vi "Main.vi"() -> ()   [LabVIEW 2013]
uses:
  ViewCtl.ctl
  GlobalV.vi
panel:
  in  "退出":bool
  in  "ViewCtl":T1
  in  "选项":enum32{"自产包装", "外购机BSJ包装", "出货", "大箱条码打印"}(tab)
  in  "料号":string
  in  "Adress":string caption="发货地址"
  in  "产品型号":u16(ring) items=["9068", "8068", "TRG80-68", "TRG80-68AW", "TRG90-68", "TRG90-68C", "TRG90-68G", "TRG90-68W", "TRG90-68CG", "TRG90-68CW", "TRG90-68GW", "TRG90-68S", "TRG80-89", "TRG90-88", "TRG90-88B", "TRG90-88C", "TRG90-88D", "TRG90-88W", "TRG90-88BW", "TRG90-88CW", "TRG90-88DW", "TRG90-03", "TRG90-03B", "TRG90-03C", "TRG90-03D", "TRG90-03E", "TRG90-03F", "TRG80-03", "TRG80-03B", "TRG80-03D"]
  out "整箱数量":string
  in  "允许未满封箱？":bool=TRUE
  in  "产品条码":string
  in  "手动装箱":bool
  in  "删除单个条码":bool
  in  "包装箱内数据":i32(listbox)
  in  "产品类别":u16(ring) items=["带卡产品", "非带卡产品"]
  in  "扫描方式":u16(ring) caption="扫描入库方式" items=["单个产品码扫描", "整箱产品码扫描"]
  out "记录导入结果":string
  in  "客户地址":string caption="发货地址"
  in  "能未满封箱？":bool=TRUE caption="允许未满封箱？"
  in  "SN码":string caption="产品条码"
  in  "人工封箱":bool
  in  "删除单个数据":bool
  in  "数据导入":bool
  in  "BSJ型号":u16(ring) caption="产品型号" items=["90-18", "90-68"]
  out "一箱数量":string
  in  "BSJ产品记录":i32(listbox)
  in  "地址":string
  in  "导出":bool
  in  "型号":u16(ring) caption="产品型号" items=["90-18", "9068"]
  in  "出货地址":string
  in  "手动出货":bool
  in  "包装箱条码":string
  in  "设定出货数量":string
  in  "出货方式":bool=TRUE
  in  "箱内产品信息":i32(listbox)
  in  "结束时间":timestamp=timestamp(3579818400.015625 s since 1904-01-01) format="%<%H:%M:%S\n%Y/%m/%d>T"
  in  "开始时间":timestamp=timestamp(3579213600.234375 s since 1904-01-01) format="%<%H:%M:%S\n%Y/%m/%d>T"
  in  "导出方式":u16(ring)=1 items=["发货地址", "包装时间", "地址和包装时间"]
  in  "产品种类":u16(ring) items=["外购带卡", "外购不带卡", "自产"]
  in  "类别":u16(ring) caption="产品种类" items=["外购", "自产"]
  in  "PModel":u16(ring) caption="产品型号" items=["9068", "8068", "TRG80-68", "TRG80-68AW", "TRG90-68", "TRG90-68C", "TRG90-68G", "TRG90-68W", "TRG90-68CG", "TRG90-68CW", "TRG90-68GW", "TRG90-68S", "TRG80-89", "TRG90-88", "TRG90-88B", "TRG90-88C", "TRG90-88D", "TRG90-88W", "TRG90-88BW", "TRG90-88CW", "TRG90-88DW", "TRG90-03", "TRG90-03B", "TRG90-03C", "TRG90-03D", "TRG90-03E", "TRG90-03F", "TRG80-03", "TRG80-03B", "TRG80-03D"]
  out "当前大箱内数量":u32
  in  "清空":bool
  in  "条码":string caption="中箱条码"
  out "大箱内产品":string
  in  "设定大箱总数":i32 step=1
  in  "手动计数打印？":bool=TRUE
  in  "手动打印":bool
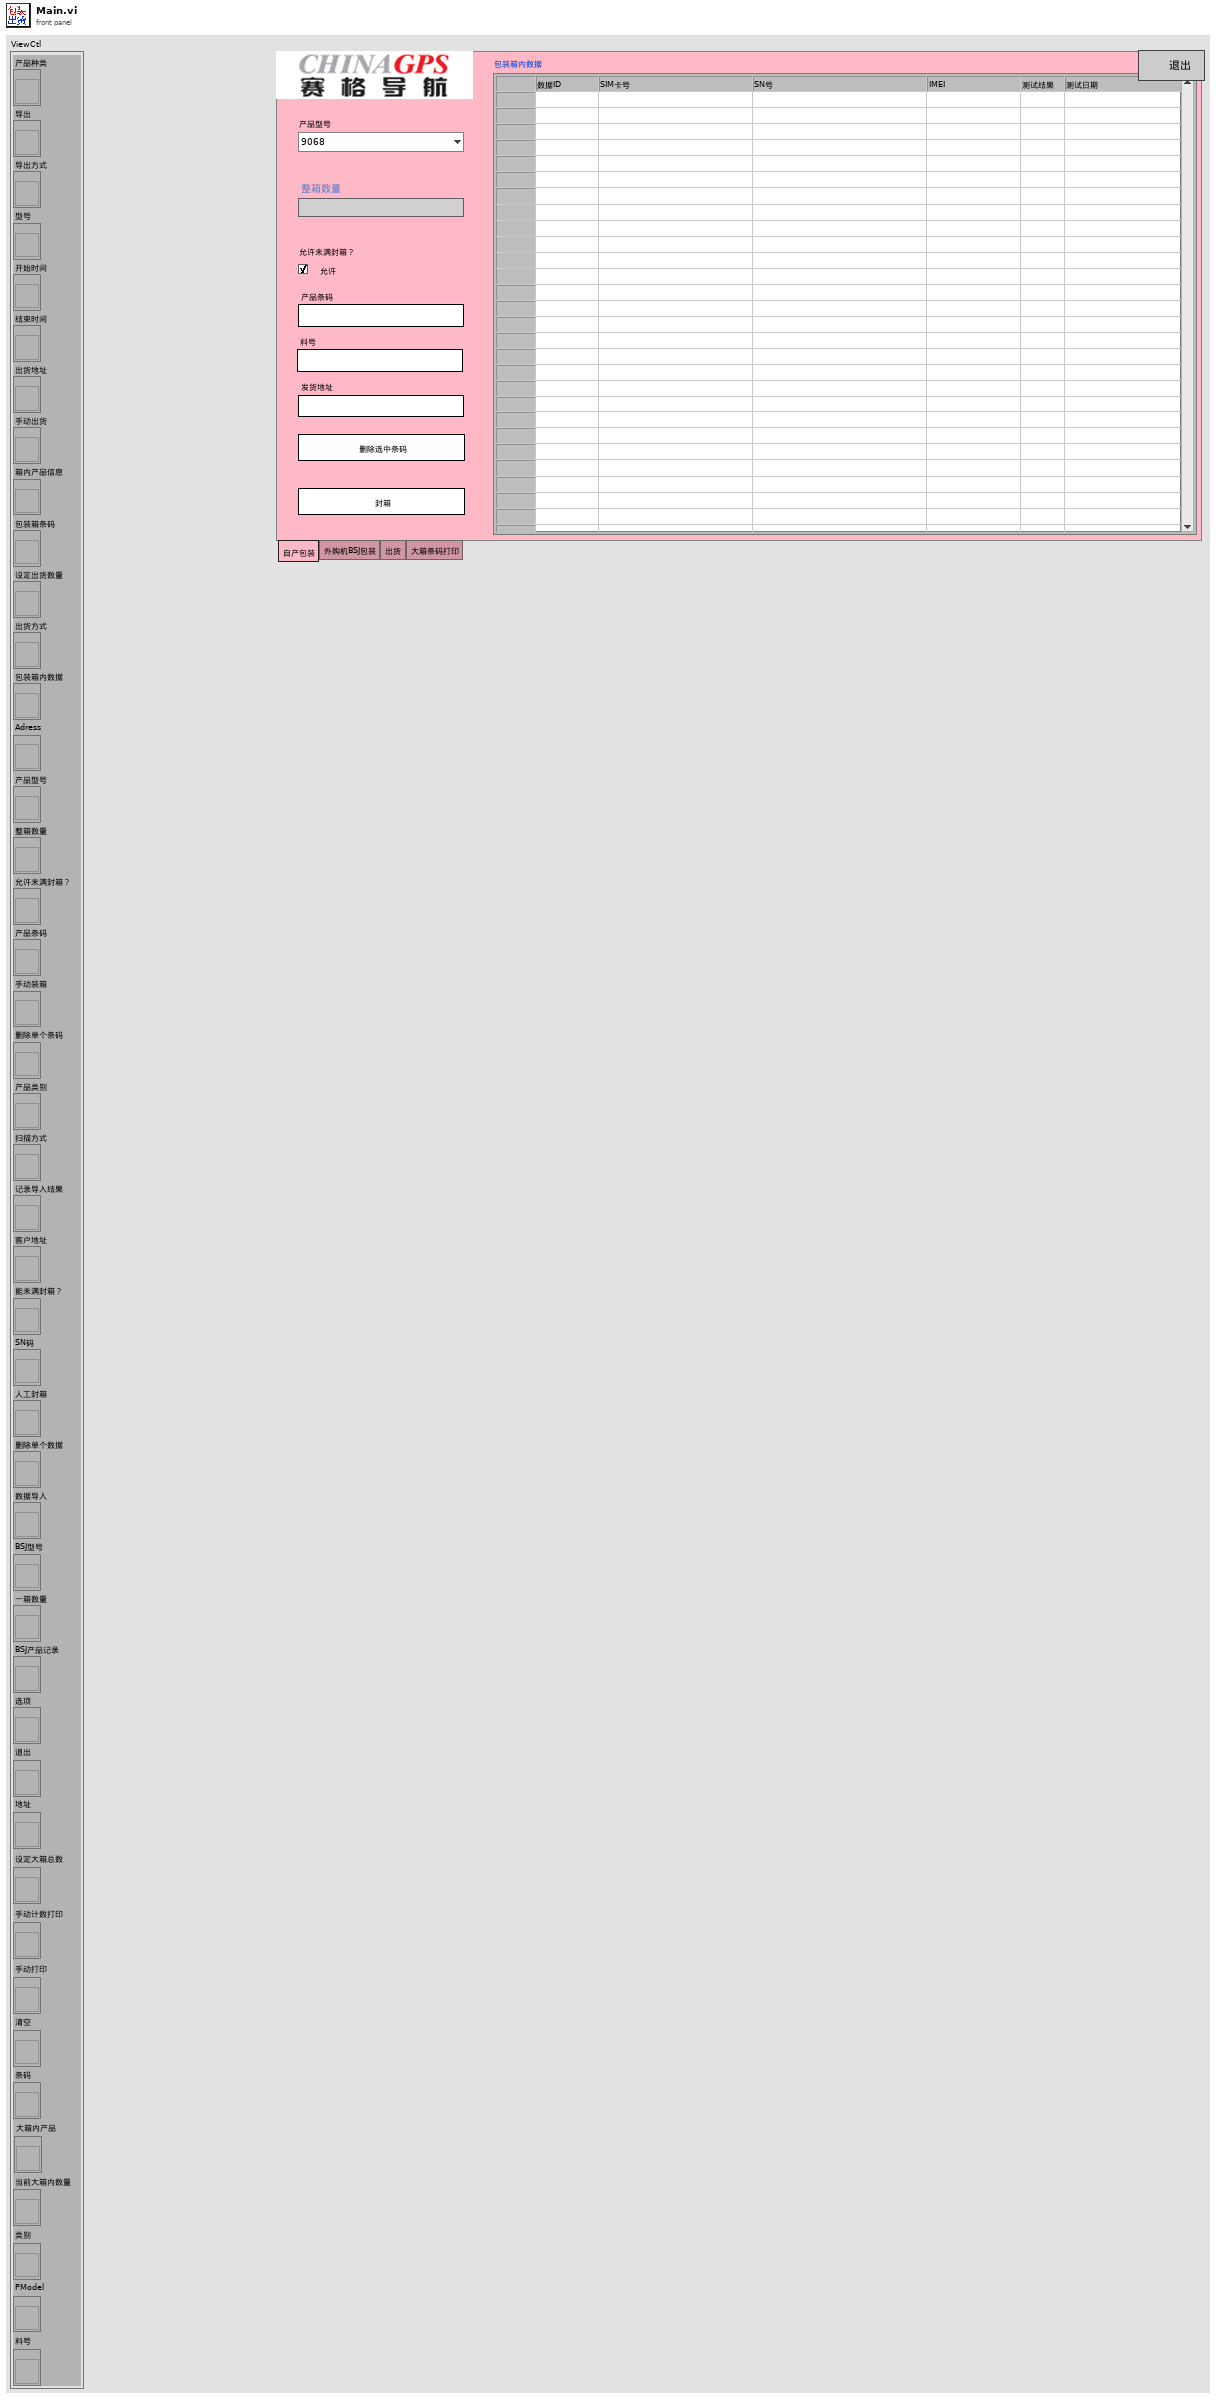
[diagram p1: front panel]
types:
  T1 = typedef "ViewCtl.ctl" = cluster{"产品种类":refnum<vi>, "导出":refnum<vi>, "导出方式":refnum<vi>, "型号":refnum<vi>, "开始时间":refnum<vi>, "结束时间":refnum<vi>, "出货地址":refnum<vi>, "手动出货":refnum<vi>, "箱内产品信息":refnum<vi>, "包装箱条码":refnum<vi>, "设定出货数量":refnum<vi>, "出货方式":refnum<vi>, "包装箱内数据":refnum<vi>, "Adress":refnum<vi>, "产品型号":refnum<vi>, "整箱数量":refnum<vi>, "允许未满封箱？":refnum<vi>, "产品条码":refnum<vi>, "手动装箱":refnum<vi>, "删除单个条码":refnum<vi>, "产品类别":refnum<vi>, "扫描方式":refnum<vi>, "记录导入结果":refnum<vi>, "客户地址":refnum<vi>, "能未满封箱？":refnum<vi>, "SN码":refnum<vi>, "人工封箱":refnum<vi>, "删除单个数据":refnum<vi>, "数据导入":refnum<vi>, "BSJ型号":refnum<vi>, "一箱数量":refnum<vi>, "BSJ产品记录":refnum<vi>, "选项":refnum<vi>, "退出":refnum<vi>, "地址":refnum<vi>, "设定大箱总数":refnum<vi>, "手动计数打印":refnum<vi>, "手动打印":refnum<vi>, "清空":refnum<vi>, "条码":refnum<vi>, "大箱内产品":refnum<vi>, "当前大箱内数量":refnum<vi>, "类别":refnum<vi>, "PModel":refnum<vi>, "料号":refnum<vi>}
  T2 = cluster{"事件注册引用句柄":refnum<event-registration>, "事件注册引用句柄":refnum<event-registration>}
  T3 = enum8{"Enabled", "Disabled", "Disabled and Grayed Out"}
  T4 = typedef "LVRowAndColumnUnsignedTypeDef.ctl" = cluster{"Row":u32, "Column":u32}
  T5 = enum32{"invalid app kind", "Development System", "Run Time System", "Student Edition", "Embedded LabVIEW", "Evaluation", "Custom"}
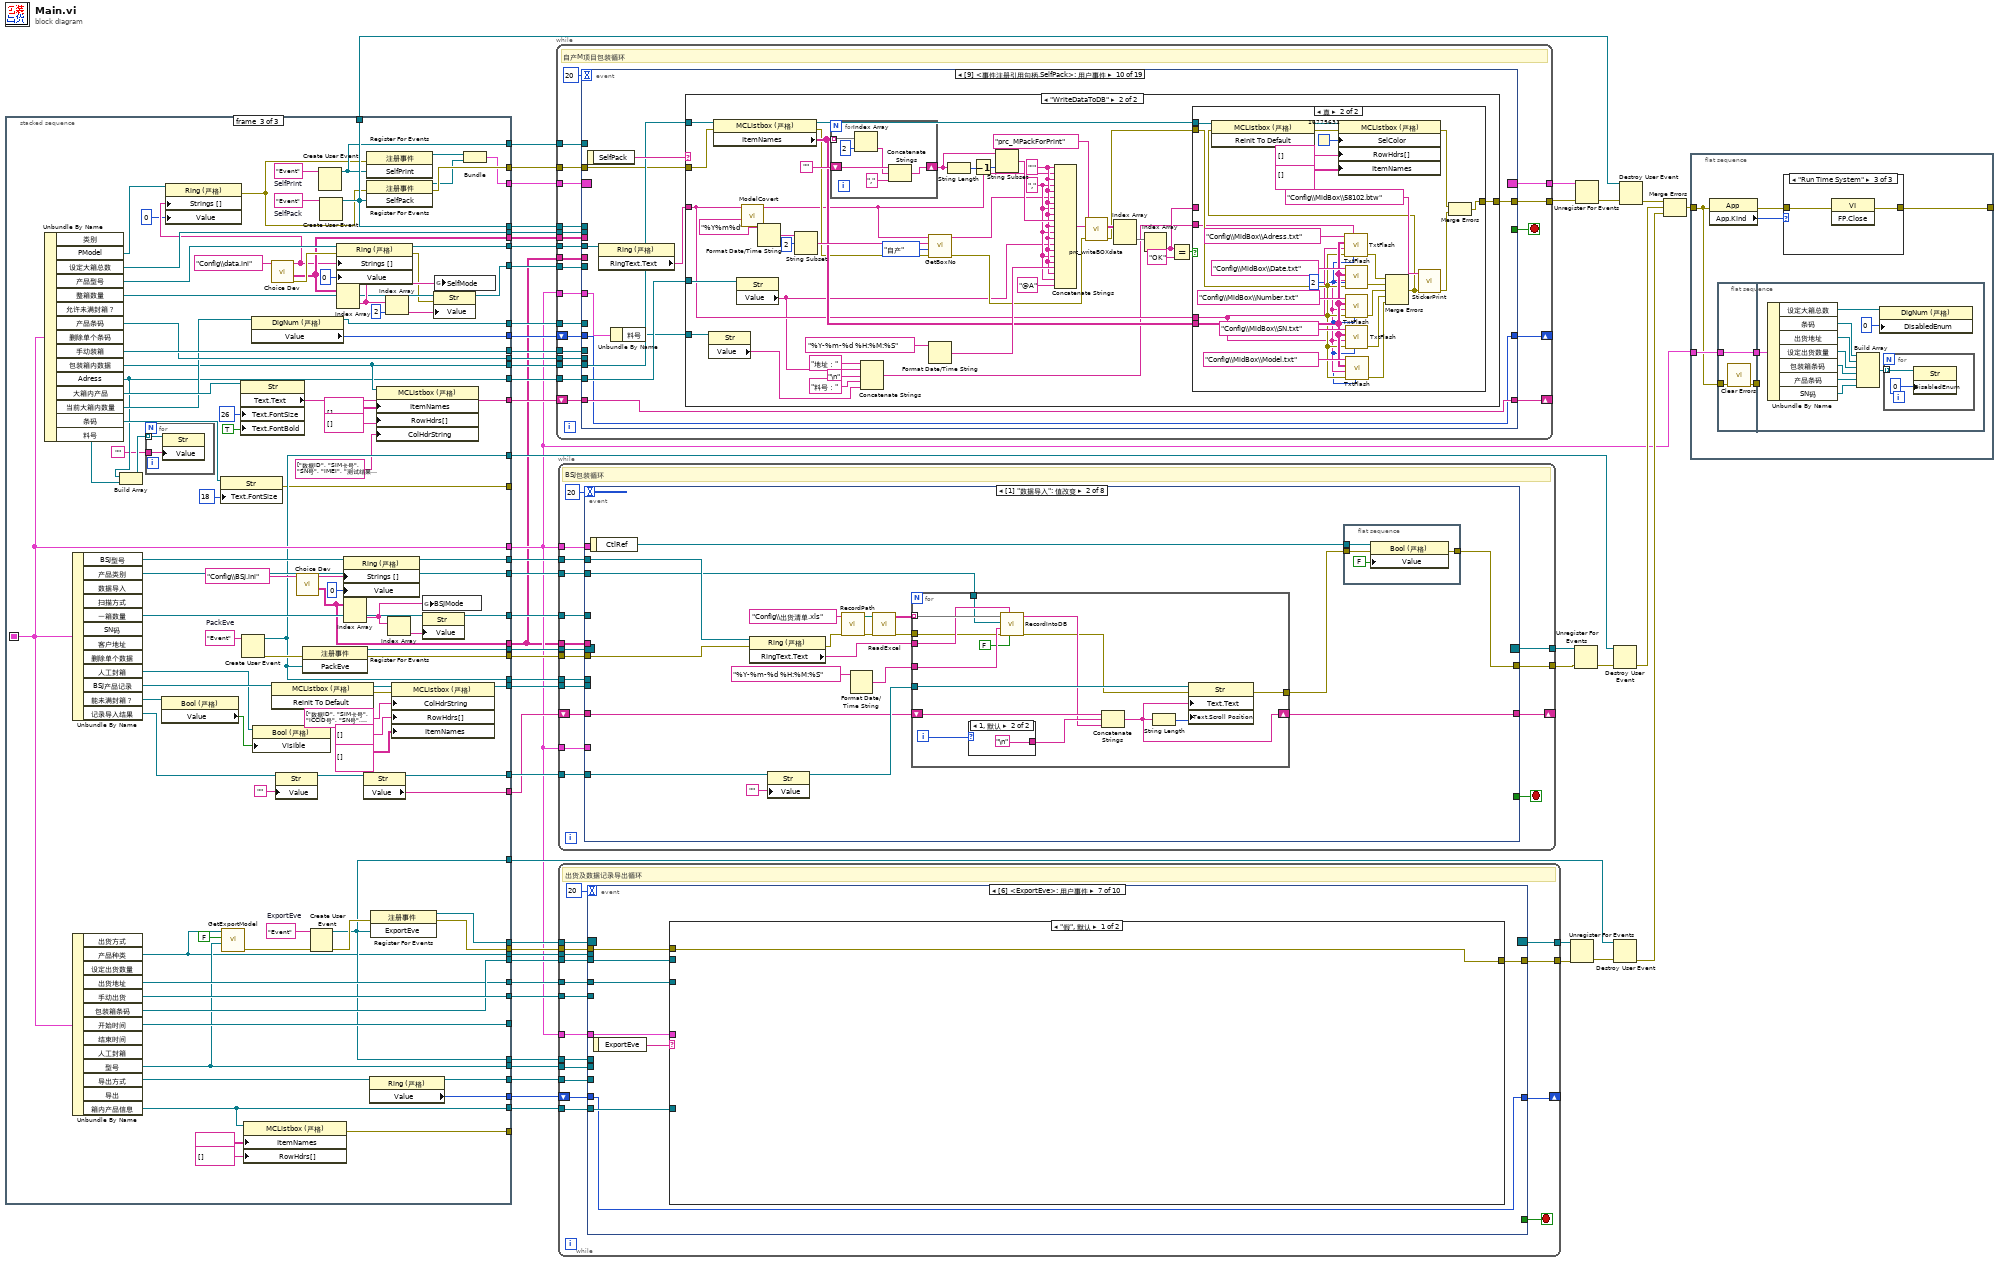
[diagram p0: block diagram]
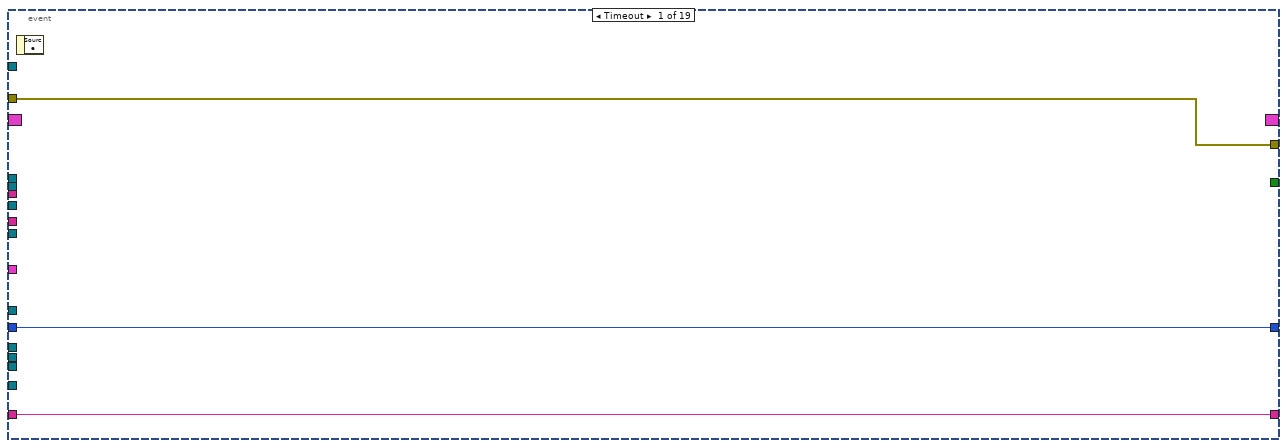
[diagram p4: hidden frame]
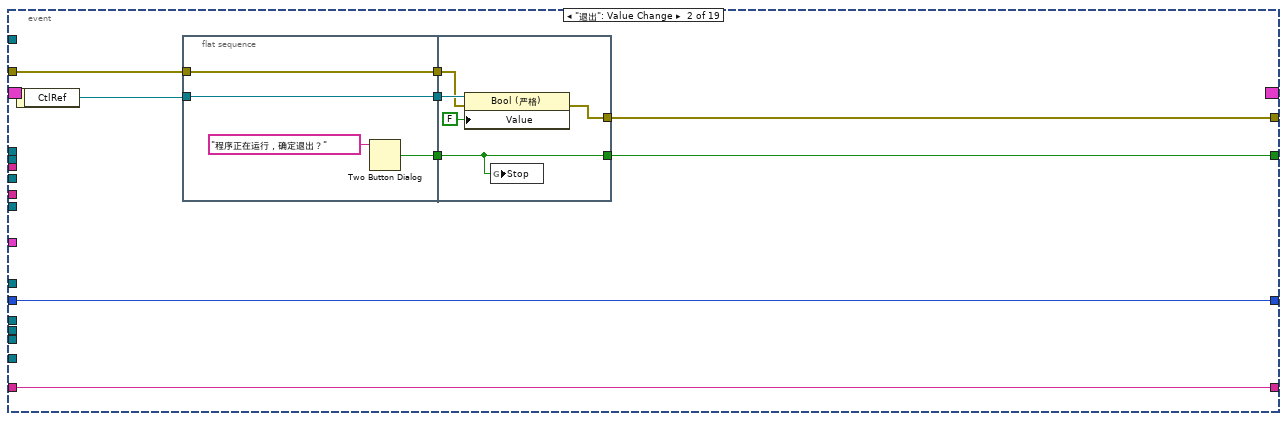
[diagram p5: hidden frame]
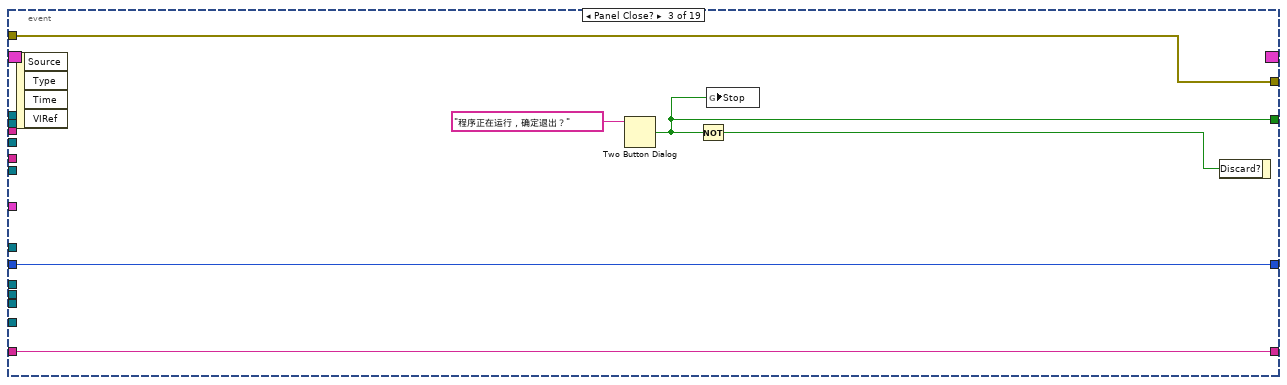
[diagram p6: hidden frame]
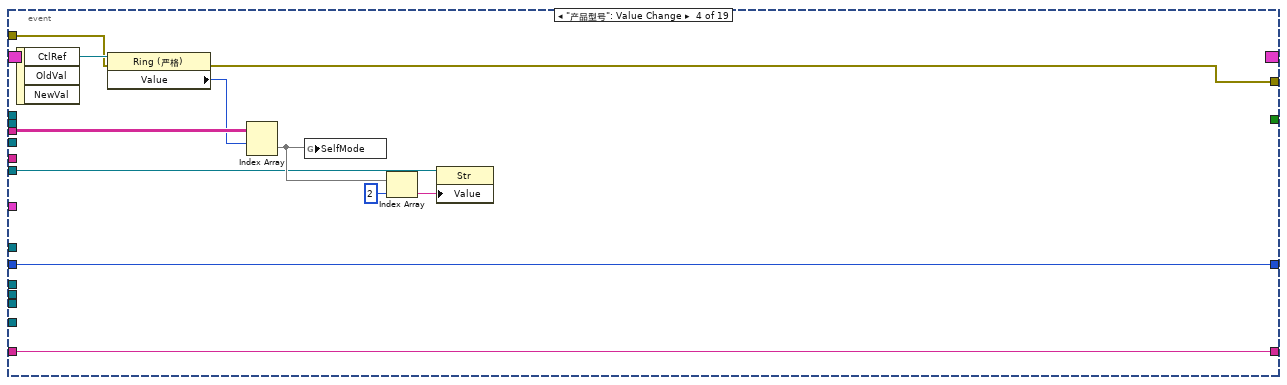
[diagram p7: hidden frame]
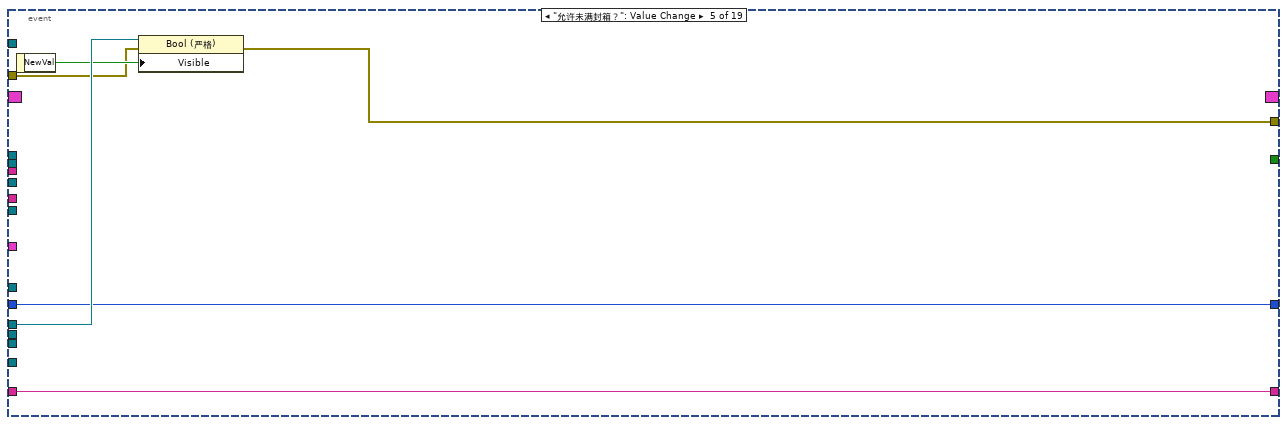
[diagram p8: hidden frame]
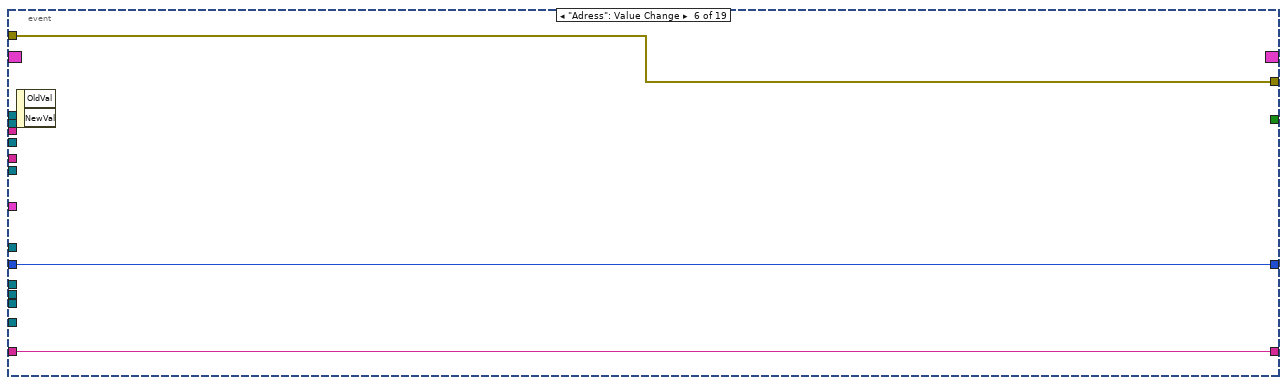
[diagram p9: hidden frame]
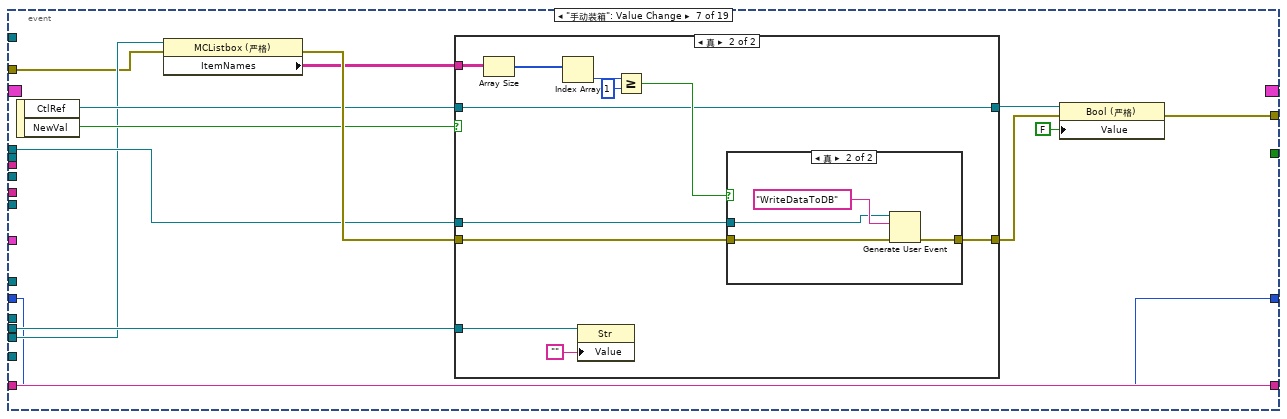
[diagram p10: hidden frame]
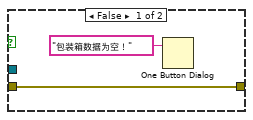
[diagram p12: hidden frame]
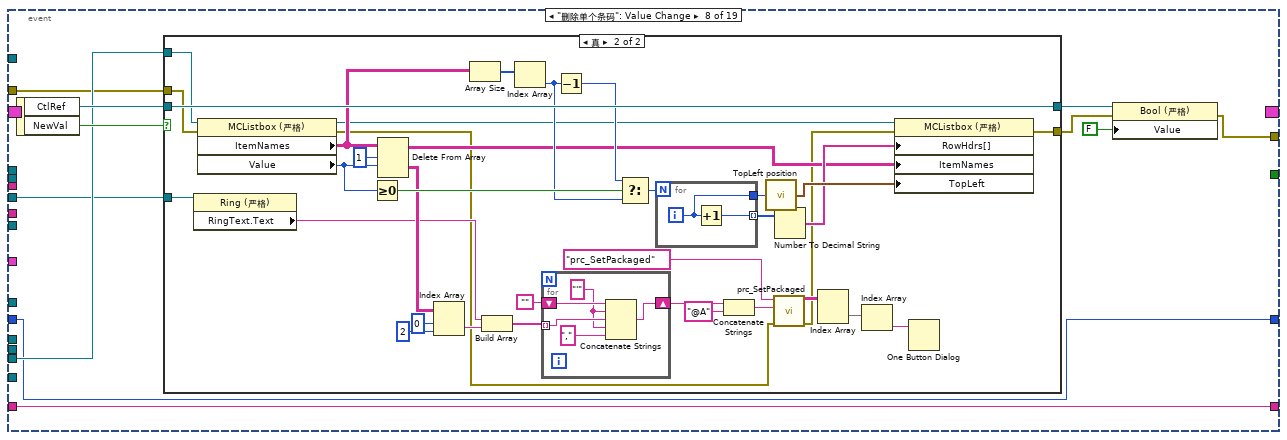
[diagram p13: hidden frame]
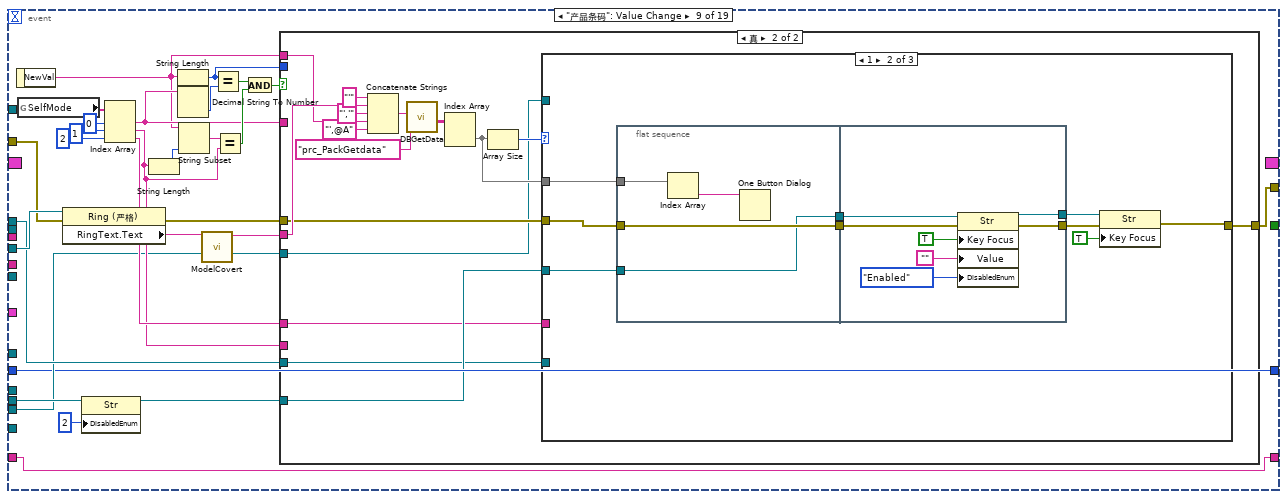
[diagram p15: hidden frame]
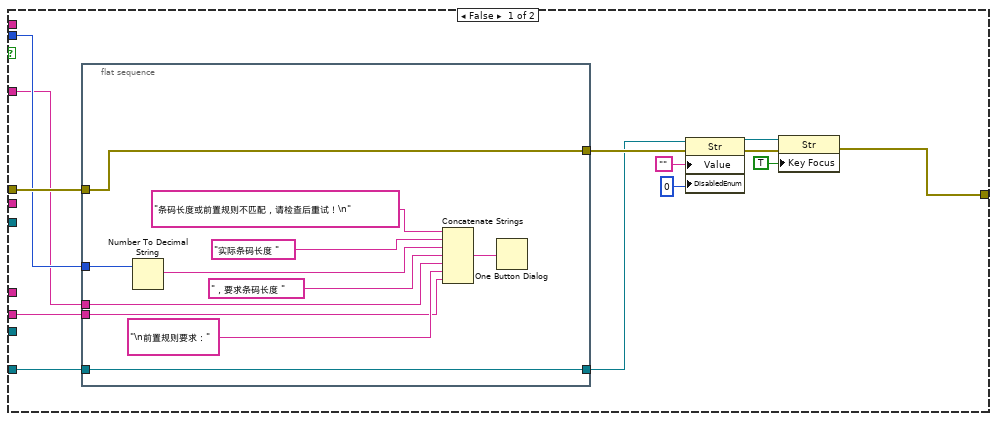
[diagram p16: hidden frame]
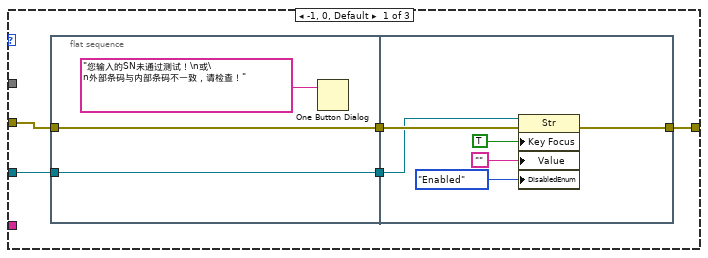
[diagram p17: hidden frame]
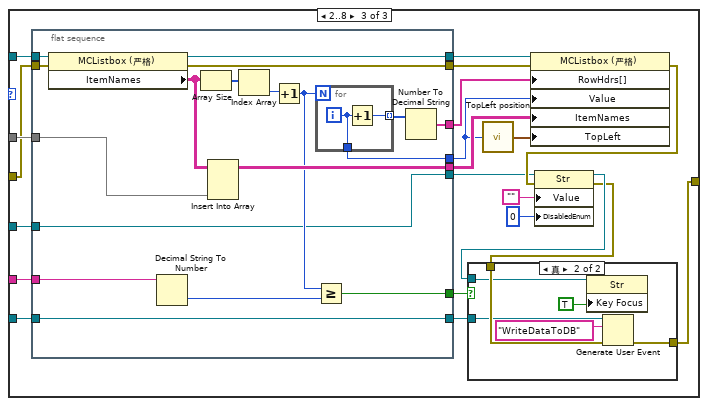
[diagram p18: hidden frame]
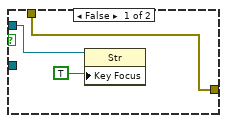
[diagram p19: hidden frame]
diagram:
  n1 = stacked-sequence {
    seq-local: [_ w57 _] -> [_ _ w175]
    tunnel: [_ _ w188] -> w45
    tunnel: [_ _ w185] -> w53
    tunnel: [_ _ w181] -> w52
    tunnel: [_ _ w180] -> w51
    tunnel: [_ _ w179] -> w50
    tunnel: [_ _ w178] -> w1
    tunnel: [_ _ w177] -> w49
    tunnel: [_ _ w176] -> w48
    tunnel: [_ _ w175] -> w3
    tunnel: [_ _ w174] -> w47
    tunnel: [_ _ w146] -> w46
    tunnel: [_ _ w173] -> w44
    tunnel: [_ _ w118] -> w43
    tunnel: [_ _ w171] -> w42
    tunnel: [_ _ w169] -> w41
    tunnel: [_ _ w117] -> w40
    tunnel: [_ _ w168] -> w39
    tunnel: [_ _ w145] -> w38
    tunnel: [_ _ w127] -> w37
    tunnel: [_ _ w167] -> w36
    tunnel: [_ _ w165] -> w35
    tunnel: [_ _ w164] -> w34
    tunnel: [_ _ w163] -> _
    tunnel: [_ _ w153] -> w33
    tunnel: [_ _ w152] -> w32
    tunnel: [_ _ w134] -> w31
    tunnel: [_ _ w147] -> w30
    tunnel: [_ _ w150] -> w29
    tunnel: [_ _ w125] -> w28
    tunnel: [_ _ w149] -> w27
    tunnel: [_ _ w111] -> w26
    tunnel: [_ _ w148] -> w22
    tunnel: [_ _ w147] -> w17
    tunnel: [_ _ w146] -> w15
    tunnel: [_ _ w145] -> w13
    tunnel: [_ _ w143] -> w8
    tunnel: [_ _ w141] -> w7
    tunnel: [_ _ w138] -> w6
    tunnel: [_ _ w133] -> w5
    tunnel: [_ _ w132] -> w4
    tunnel: [_ _ w129] -> _
    tunnel: [_ _ w128] -> w2
    tunnel: [_ _ w120] -> _
    frame #0 {
      n2 = global write "GlobalV.vi" "Stop"(FALSE ("Stop")) -> ()
    }
    frame #1 {
      n3 = invoke class="VI" method="Default Vals.Reinit All"() -> (error out=w58:errorcluster)  [unwired: 3 in, 2 out]
      n4 = flat-sequence {
        tunnel: w58 -> [_]
        tunnel: [w73] -> w57
        frame #0 {
          n5 = control-ref of="箱内产品信息"() -> (w98:refnum<vi>)
          n6 = control-ref of="包装箱内数据"() -> (w94:refnum<vi>)
          n7 = control-ref of="BSJ产品记录"() -> (w75:refnum<vi>)
          n8 = control-ref of="选项"() -> (w74:refnum<vi>)
          n9 = control-ref of="产品种类"() -> (w106:refnum<vi>)
          n10 = control-ref of="导出方式"() -> (w104:refnum<vi>)
          n11 = control-ref of="型号"() -> (w103:refnum<vi>)
          n12 = control-ref of="开始时间"() -> (w102:refnum<vi>)
          n13 = control-ref of="结束时间"() -> (w101:refnum<vi>)
          n14 = control-ref of="产品型号"() -> (w92:refnum<vi>)
          n15 = control-ref of="产品类别"() -> (w86:refnum<vi>)
          n16 = control-ref of="扫描方式"() -> (w85:refnum<vi>)
          n17 = control-ref of="BSJ型号"() -> (w77:refnum<vi>)
          n18 = control-ref of="类别"() -> (w63:refnum<vi>)
          n19 = control-ref of="PModel"() -> (w62:refnum<vi>)
          n20 = control-ref of="出货地址"() -> (w100:refnum<vi>)
          n21 = control-ref of="包装箱条码"() -> (w97:refnum<vi>)
          n22 = control-ref of="设定出货数量"() -> (w96:refnum<vi>)
          n23 = control-ref of="Adress"() -> (w93:refnum<vi>)
          n24 = control-ref of="整箱数量"() -> (w91:refnum<vi>)
          n25 = control-ref of="产品条码"() -> (w89:refnum<vi>)
          n26 = control-ref of="记录导入结果"() -> (w84:refnum<vi>)
          n27 = control-ref of="客户地址"() -> (w83:refnum<vi>)
          n28 = control-ref of="SN码"() -> (w81:refnum<vi>)
          n29 = control-ref of="一箱数量"() -> (w76:refnum<vi>)
          n30 = control-ref of="地址"() -> (w71:refnum<vi>)
          n31 = control-ref of="条码"() -> (w66:refnum<vi>)
          n32 = control-ref of="大箱内产品"() -> (w65:refnum<vi>)
          n33 = control-ref of="料号"() -> (w61:refnum<vi>)
          n34 = control-ref of="导出"() -> (w105:refnum<vi>)
          n35 = control-ref of="手动出货"() -> (w99:refnum<vi>)
          n36 = control-ref of="出货方式"() -> (w95:refnum<vi>)
          n37 = control-ref of="允许未满封箱？"() -> (w90:refnum<vi>)
          n38 = control-ref of="手动装箱"() -> (w88:refnum<vi>)
          n39 = control-ref of="删除单个条码"() -> (w87:refnum<vi>)
          n40 = control-ref of="能未满封箱？"() -> (w82:refnum<vi>)
          n41 = control-ref of="人工封箱"() -> (w80:refnum<vi>)
          n42 = control-ref of="删除单个数据"() -> (w79:refnum<vi>)
          n43 = control-ref of="数据导入"() -> (w78:refnum<vi>)
          n44 = control-ref of="退出"() -> (w72:refnum<vi>)
          n45 = control-ref of="设定大箱总数"() -> (w70:refnum<vi>)
          n46 = control-ref of="手动计数打印？"() -> (w69:refnum<vi>)
          n47 = control-ref of="手动打印"() -> (w68:refnum<vi>)
          n48 = control-ref of="清空"() -> (w67:refnum<vi>)
          n49 = control-ref of="当前大箱内数量"() -> (w64:refnum<vi>)
          n50 = Bundle By Name(cluster="ViewCtl", "产品种类"=w106, "导出"=w105, "导出方式"=w104, "型号"=w103, "开始时间"=w102, "结束时间"=w101, "出货地址"=w100, "手动出货"=w99, "箱内产品信息"=w98, "包装箱条码"=w97, "设定出货数量"=w96, "出货方式"=w95, "包装箱内数据"=w94, "Adress"=w93, "产品型号"=w92, "整箱数量"=w91, "允许未满封箱？"=w90, "产品条码"=w89, "手动装箱"=w88, "删除单个条码"=w87, "产品类别"=w86, "扫描方式"=w85, "记录导入结果"=w84, "客户地址"=w83, "能未满封箱？"=w82, "SN码"=w81, "人工封箱"=w80, "删除单个数据"=w79, "数据导入"=w78, "BSJ型号"=w77, "一箱数量"=w76, "BSJ产品记录"=w75, "选项"=w74, "退出"=w72, "地址"=w71, "设定大箱总数"=w70, "手动计数打印"=w69, "手动打印"=w68, "清空"=w67, "条码"=w66, "大箱内产品"=w65, "当前大箱内数量"=w64, "类别"=w63, "PModel"=w62, "料号"=w61) -> (w73:T1)
        }
      }
      n51 = Unbundle By Name(w57) -> ("选项"=w56:refnum<vi>)
      n52 = property class="TabCtl (严格)"(reference=w56) -> ("Pages"=w55:refnum<vi>[])  [unwired: 1 in, 2 out]
      n53 = for {
        tunnel: w55 -> [w60] mode=indexing
        n54 = property class="Page"(reference=w60, "PageEnb"=2) -> ()  [unwired: 1 in, 2 out]
      }
    }
    frame #2 {
      w137 = "Event"  # SelfPrint
      w151 = "Event"  # SelfPack
      w172 = "Event"  # ExportEve
      w187 = "Event"  # PackEve
      n55 = Unbundle By Name(w175) -> ("PModel"=w115:refnum<vi>, "设定大箱总数"=w138:refnum<vi>, "产品型号"=w161:refnum<vi>, "整箱数量"=w158:refnum<vi>, "产品条码"=w150:refnum<vi>, "手动装箱"=w152:refnum<vi>, "包装箱内数据"=w125:refnum<vi>, "Adress"=w111:refnum<vi>, "大箱内产品"=w144:refnum<vi>, "当前大箱内数量"=w142:refnum<vi>, "条码"=w131:refnum<vi>, "料号"=w110:refnum<vi>)  [unwired: 3 out]
      n56 = Unbundle By Name(w175) -> ("BSJ型号"=w203:refnum<vi>, "产品类别"=w174:refnum<vi>, "一箱数量"=w192:refnum<vi>, "人工封箱"=w190:refnum<vi>, "BSJ产品记录"=w200:refnum<vi>, "能未满封箱？"=w191:refnum<vi>, "记录导入结果"=w183:refnum<vi>)  [unwired: 5 out]
      n57 = Unbundle By Name(w175) -> ("产品种类"=w117:refnum<vi>, "出货地址"=w167:refnum<vi>, "手动出货"=w173:refnum<vi>, "包装箱条码"=w168:refnum<vi>, "开始时间"=w163:refnum<vi>, "型号"=w118:refnum<vi>, "导出方式"=w166:refnum<vi>, "箱内产品信息"=w127:refnum<vi>)  [unwired: 5 out]
      n58 = Build Array(w111, w110) -> (w109:refnum<vi>[])
      n59 = for {
        tunnel: w109 -> [w206] mode=indexing
        tunnel: "" -> [w205]
        n60 = property class="Str"(reference=w206, "Value"=w205) -> ()  [unwired: 1 in, 2 out]
      }
      n61 = property class="Bool (严格)"(reference=w191) -> ("Value"=w189:bool)  [unwired: 1 in, 2 out]
      n62 = property class="Str"(reference=w131, "Text.FontSize"=u32 18 ("文本.字体:字号")) -> (error out=w129:errorcluster)  [unwired: 1 in, 1 out]
      n63 = call "GetExportModel.vi"("型号"=w118, "Debug"=FALSE, "产品类型"=w117) -> ("error out"=w116:errorcluster)  [unwired: 8 in]
      n64 = property class="Str"(reference=w144, "Text.FontSize"=u32 26 ("文本.字体:字号"), "Text.FontBold"=TRUE) -> ("Text.Text"=w143:string)  [unwired: 1 in, 2 out]
      n65 = Create User Event(user event datatype=w187) -> (user event=w146:refnum<user-event>, error out=w186:errorcluster)  [unwired: 1 in]
      n66 = property class="MCListbox (严格)"(reference=w127, "ItemNames"=string[][] [] ("项名"), "RowHdrs[]"=string[] [] ("行首字符串[]")) -> (error out=w120:errorcluster)  [unwired: 1 in, 1 out]
      n67 = property class="DigNum (严格)"(reference=w142) -> (reference out=w132:refnum<vi>, "Value"=w141:u32)  [unwired: 1 in, 1 out]
      n68 = property class="Bool (严格)"(reference=w190, "Visible"=w189) -> ()  [unwired: 1 in, 2 out]
      n69 = call "Choice Dev.vi"("Path"="Config\\data.ini") -> ("error out"=w155:errorcluster, "data"=w153:string[][], "model"=w114:string[])  [unwired: 7 in]
      n70 = property class="Ring (严格)"(reference=w115, "Strings []"=w114, "Value"=u16 0 ("值")) -> (error out=w112:errorcluster)  [unwired: 1 in, 1 out]
      n71 = invoke class="MCListbox (严格)" method="Reinit To Default"(reference=w200) -> (reference out=w199:refnum<vi>, error out=w195:errorcluster)  [unwired: 2 in, 1 out]
      n72 = property class="Str"(reference=w183, "Value"="") -> (reference out=w182:refnum<vi>)  [unwired: 1 in, 1 out]
      n73 = call "Choice Dev.vi"("Path"="Config\\BSJ.ini") -> ("data"=w178:string[][], "model"=w202:string[])  [unwired: 7 in, 1 out]
      n74 = register-events(error in=w186, w146) -> (reference out=w185:refnum<event-registration>, error out=w176:errorcluster)  [unwired: 1 in]
      n75 = Create User Event(user event datatype=w172, error in=w116) -> (user event=w145:refnum<user-event>, error out=w170:errorcluster)
      n76 = Create User Event(user event datatype=w137) -> (user event=w133:refnum<user-event>)  [unwired: 1 in, 1 out]
      n77 = Create User Event(user event datatype=w151) -> (user event=w147:refnum<user-event>)  [unwired: 1 in, 1 out]
      n78 = property class="Ring (严格)"(reference=w161, error in=w155, "Strings []"=w114, "Value"=u16 0 ("值")) -> (reference out=w149:refnum<vi>, error out=w154:errorcluster)
      n79 = Index Array(array=w153) -> (element=w159:string[])  [unwired: 2 in]
      n80 = property class="Ring (严格)"(reference=w203, "Strings []"=w202, "Value"=u16 0 ("值")) -> (reference out=w179:refnum<vi>)  [unwired: 1 in, 1 out]
      n81 = Index Array(array=w178) -> (element=w194:string[])  [unwired: 2 in]
      n82 = property class="Str"(reference=w182) -> (reference out=w181:refnum<vi>, "Value"=w180:string)  [unwired: 1 in, 1 out]
      n83 = register-events(error in=w112, w133) -> (reference out=w136:refnum<event-registration>)  [unwired: 1 in, 1 out]
      n84 = register-events(error in=w112, w147) -> (reference out=w135:refnum<event-registration>, error out=w148:errorcluster)  [unwired: 1 in]
      n85 = property class="Ring (严格)"(reference=w166) -> (reference out=w164:refnum<vi>, "Value"=w165:u16)  [unwired: 1 in, 1 out]
      n86 = register-events(error in=w170, w145) -> (reference out=w171:refnum<event-registration>, error out=w169:errorcluster)  [unwired: 1 in]
      n87 = property class="MCListbox (严格)"(reference=w125, "ItemNames"=string[][] [] ("项名"), "RowHdrs[]"=string[] [] ("行首字符串[]"), "ColHdrString"=string[] ["数据ID", "SIM卡号", "SN号", "IMEI", "测试结果", "测试日期"]) -> ()  [unwired: 1 in, 2 out]
      n88 = Index Array(array=w159, index=2 ("索引")) -> (element=w157:string)
      n89 = Index Array(array=w194) -> (element=w193:string)  [unwired: 1 in]
      n90 = property class="MCListbox (严格)"(reference=w199, error in=w195, "ColHdrString"=string[] ["数据ID", "SIM卡号", "ICCID号", "SN号", "导入日期"], "RowHdrs[]"=string[] [] ("行首字符串[]"), "ItemNames"=string[][] [] ("项名")) -> (reference out=w188:refnum<vi>)  [unwired: 1 out]
      n91 = global write "GlobalV.vi" "BSJMode"(w194) -> ()
      n92 = property class="Str"(reference=w192, "Value"=w193) -> (reference out=w177:refnum<vi>)  [unwired: 1 in, 1 out]
      n93 = property class="Str"(reference=w158, error in=w154, "Value"=w157) -> (reference out=w128:refnum<vi>)  [unwired: 1 out]
      n94 = global write "GlobalV.vi" "SelfMode"(w159) -> ()
      n95 = Bundle("事件注册引用句柄"=w136, "事件注册引用句柄"=w135) -> (w134:T2)  [unwired: 1 in]
    }
  }
  n96 = while {
    tunnel: w33 -> [w227]
    tunnel: w32 -> [w226]
    tunnel: w31 -> [w225]
    tunnel: w30 -> [w224]
    tunnel: w29 -> [w223]
    tunnel: w28 -> [w222]
    tunnel: w27 -> [w221]
    tunnel: w26 -> [w220]
    tunnel: [w219] -> w25
    tunnel: w22 -> [w218]
    tunnel: [w217] -> w21
    tunnel: w3 -> [w216]
    shift-right: [w214] -> _
    shift-left: w8 -> [w215]
    shift-right: [w212] -> _
    shift-left: w7 -> [w213]
    tunnel: w6 -> [w211]
    tunnel: w5 -> [w210]
    tunnel: w4 -> [w209]
    tunnel: w2 -> [w208]
    tunnel: w1 -> [w207]
    stop <- w228 stop-if-true
    # "自产M项目包装循环"
    n97 = event shown="[9] <事件注册引用句柄.SelfPack>: 用户事件" {
      selector: w225 -> [_ _ _ _ _ _ _ _ _ _ _ _ _ _ _ _ _ _ _]
      dyn-events: [_ _ _ _ _ _ _ _ _ _ _ _ _ _ _ _ _ _ _] -> w219
      timeout: 20 -> [_ _ _ _ _ _ _ _ _ _ _ _ _ _ _ _ _ _ _]
      tunnel: [_ w238 w254 _ _ _ _ _ _ _ _ _ _ _ _ _ _ _ _] -> w228
      tunnel: w227 -> [_ _ _ w266 _ _ _ _ _ _ _ _ _ _ _ _ _ w1126 _]
      tunnel: w226 -> [_ _ _ _ w273 _ _ _ _ _ _ _ _ _ _ _ _ _ _]
      tunnel: w224 -> [_ _ _ _ _ _ w283 _ w376 _ _ _ _ _ _ _ _ _ _]
      tunnel: w223 -> [_ _ _ _ _ _ w282 _ w381 _ _ _ _ _ _ _ _ _ _]
      tunnel: w222 -> [_ _ _ _ _ _ w281 w316 w372 w526 _ _ _ _ _ _ _ _ _]
      tunnel: w221 -> [_ _ _ _ _ _ _ w315 w378 w525 _ _ _ _ _ _ _ _ _]
      tunnel: w220 -> [_ _ _ _ _ _ _ _ _ w523 _ _ _ _ _ _ _ _ _]
      tunnel: w218 -> [w232 w236 w253 w264 w271 w276 w280 w313 w371 w522 w608 w752 w796 w805 w1012 w1044 w1098 w1134 w1148]
      tunnel: [w232 w235 w253 w263 w270 w276 w279 w312 w370 w521 w608 w751 w795 w806 w1006 w1043 w1097 w1134 w1148] -> w217
      tunnel: w216 -> [_ _ _ _ _ _ _ _ _ w518 w606 _ w799 w817 _ w1040 w1100 w1131 w1139]
      tunnel: w215 -> [w231 w234 w252 w262 w269 w275 w278 w311 w369 w520 w605 w750 w794 w800 w1011 w1038 w1103 w1133 w1145]
      tunnel: [w231 w234 w252 w262 w269 w275 w278 w311 w369 w520 w605 w750 w794 w807 w1011 w1039 w1103 w1133 w1140] -> w214
      tunnel: w213 -> [w230 w233 w251 w261 w268 w274 w277 w310 w368 w519 w604 w749 w793 w820 w1013 w1037 w1102 w1132 w1144]
      tunnel: [w230 w233 w251 w261 w268 w274 w277 w310 w368 w519 w604 w749 w793 w819 w1013 w1036 w1102 w1132 w1141] -> w212
      tunnel: w211 -> [_ _ _ _ _ _ _ _ _ _ _ _ _ w810 _ _ _ _ _]
      tunnel: w210 -> [_ _ _ _ _ _ _ _ _ _ _ _ _ w811 w1007 _ _ _ _]
      tunnel: w209 -> [_ _ _ _ _ _ _ _ _ _ _ _ _ w808 _ _ _ _ _]
      tunnel: w208 -> [_ _ _ w259 _ _ _ _ _ _ _ _ _ _ _ _ _ _ _]
      tunnel: w207 -> [_ _ _ _ _ _ _ _ _ _ _ _ _ _ _ _ _ w1125 _]
      event Timeout {
        n98 = event-data() -> ()  [unwired: 1 in, 1 out]
      }
      event "退出": Value Change {
        n99 = event-data() -> ("CtlRef"=w239:refnum<vi>)  [unwired: 1 in]
        n100 = flat-sequence {
          tunnel: [w244] -> w241
          tunnel: [w243] -> w240
          tunnel: w239 -> [w243]
          tunnel: [w242] -> w237
          tunnel: w236 -> [w242]
          tunnel: [w248] -> w238
          tunnel: w241 -> [w248]
          tunnel: w240 -> [w250]
          tunnel: w237 -> [w247]
          tunnel: [w246] -> w235
          frame #0 {
            n101 = Two Button Dialog(message="程序正在运行，确定退出？" ("消息")) -> (T button?=w244:bool)  [unwired: 2 in]
          }
          frame #1 {
            n102 = property class="Bool (严格)"(reference=w250, error in=w247, "Value"=FALSE) -> (error out=w246:errorcluster)  [unwired: 1 out]
            n103 = global write "GlobalV.vi" "Stop"(w248) -> ()
          }
        }
      }
      event Panel Close? {
        n104 = event-data() -> ()  [unwired: 1 in, 4 out]
        n105 = Two Button Dialog(message="程序正在运行，确定退出？" ("消息")) -> (T button?=w254:bool)  [unwired: 2 in]
        n106 = Not(x=w254) -> (.not. x?=w255:bool)
        n107 = global write "GlobalV.vi" "Stop"(w254) -> ()
        n108 = event-data("Discard?"=w255) -> ()  [unwired: 1 in, 1 out]
      }
      event "产品型号": Value Change {
        n109 = event-data() -> ("CtlRef"=w267:refnum<vi>)  [unwired: 1 in, 2 out]
        n110 = property class="Ring (严格)"(reference=w267, error in=w264) -> (error out=w263:errorcluster, "Value"=w265:u16)  [unwired: 1 out]
        n111 = Index Array(array=w266, index (row)=w265) -> (element=w260:string[])  [unwired: 1 in]
        n112 = global write "GlobalV.vi" "SelfMode"(w260) -> ()
        n113 = Index Array(array=w260, index=2 ("索引")) -> (element=w258:string)
        n114 = property class="Str"(reference=w259, "Value"=w258) -> ()  [unwired: 1 in, 2 out]
      }
      event "允许未满封箱？": Value Change {
        n115 = event-data() -> ("NewVal"=w272:bool)  [unwired: 1 in]
        n116 = property class="Bool (严格)"(reference=w273, error in=w271, "Visible"=w272) -> (error out=w270:errorcluster)  [unwired: 1 out]
      }
      event "Adress": Value Change {
        n117 = event-data() -> ()  [unwired: 1 in, 2 out]
      }
      event "手动装箱": Value Change {
        n118 = event-data() -> ("CtlRef"=w285:refnum<vi>, "NewVal"=w284:bool)  [unwired: 1 in]
        n119 = property class="MCListbox (严格)"(reference=w281, error in=w280) -> (error out=w289:errorcluster, "ItemNames"=w286:string[][])  [unwired: 1 out]
        n120 = case shown="真" w284 {
          tunnel: w285 -> [w292 w296]
          tunnel: w286 -> [_ w303]
          tunnel: w283 -> [_ w298]
          tunnel: w282 -> [_ w297]
          tunnel: [w292 w296] -> w288
          tunnel: w289 -> [w291 w295]
          tunnel: [w291 w294] -> w290
          frame False {
          }
          frame True {
            n121 = Array Size(array=w303) -> (size(s)=w302:i32[])
            n122 = Index Array(array=w302) -> (element=w301:i32)  [unwired: 1 in]
            n123 = property class="Str"(reference=w297, "Value"="") -> ()  [unwired: 1 in, 2 out]
            n124 = Greater Or Equal?(x=w301, y=1) -> (x >= y?=w299:bool)
            n125 = case shown="真" w299 {
              tunnel: w298 -> [_ w306]
              tunnel: w295 -> [w304 w308]
              tunnel: [w304 w307] -> w294
              frame False {
                n126 = One Button Dialog(message="包装箱数据为空！" ("消息")) -> ()  [unwired: 1 in, 1 out]
              }
              frame True {
                n127 = Generate User Event(user event=w306, event data cluster="WriteDataToDB" ("事件数据"), error in=w308) -> (error out=w307:errorcluster)  [unwired: 1 in, 1 out]
              }
            }
          }
        }
        n128 = property class="Bool (严格)"(reference=w288, error in=w290, "Value"=FALSE ("值")) -> (error out=w279:errorcluster)  [unwired: 1 out]
      }
      event "删除单个条码": Value Change {
        n129 = event-data() -> ("CtlRef"=w318:refnum<vi>, "NewVal"=w317:bool)  [unwired: 1 in]
        n130 = case shown="真" w317 {
          tunnel: w318 -> [w322 w357]
          tunnel: [w322 w357] -> w320
          tunnel: w316 -> [_ w356]
          tunnel: w315 -> [_ w340]
          tunnel: w313 -> [w321 w326]
          tunnel: [w321 w323] -> w314
          frame False {
          }
          frame True {
            n131 = property class="Ring (严格)"(reference=w340) -> ("RingText.Text"=w338:string)  [unwired: 1 in, 2 out]
            n132 = property class="MCListbox (严格)"(reference=w356, error in=w326) -> (reference out=w345:refnum<vi>, error out=w325:errorcluster, "ItemNames"=w354:string[][], "Value"=w352:i32)
            n133 = Greater Or Equal To 0?(x=w352) -> (x >= 0?=w351:bool)
            n134 = Delete From Array(array=w354, length=1 ("长度"), index (row)=w352) -> (deleted portion=w339:string[][], array with subset deleted=w342:string[][])  [unwired: 1 in]
            n135 = Index Array(array=w339, index (row)=0 ("索引 (行)"), index (col)=2 ("禁用的索引 (列)")) -> (element=w337:string)
            n136 = Array Size(array=w354) -> (size(s)=w353:i32[])
            n137 = Build Array(w338, w337) -> (w334:string[])
            n138 = Index Array(array=w353) -> (element=w349:i32)  [unwired: 1 in]
            n139 = for {
              tunnel: w334 -> [w361] mode=indexing
              shift-right: [w358] -> w331
              shift-left: "" -> [w362]
              w360 = "'" ("字符串")
              n140 = Concatenate Strings(w362, w360, w361, w360, "," ("字符串")) -> (w358:string)
            }
            n141 = Decrement(x=w349) -> (x-1=w350:i32)
            n142 = Select(t=w350, s=w351, f=w349) -> (s? t:f=w348:i32)
            n143 = for {
              N: w348 -> [_]
              tunnel: [w364] -> w346 mode=indexing
              tunnel: [w363] -> w347
              i -> [w363]
              n144 = Increment(x=w363) -> (x+1=w364:i32)
            }
            n145 = Concatenate Strings(w331, "@A" ("字符串")) -> (w333:string)
            n146 = call "TopLeft position.vi"("index"=w347) -> ("TopLeft"=w344:T4)
            n147 = call "prc_SetPackaged.vi"("error in"=w325, "string"=w333, "SQL query"="prc_SetPackaged") -> ("error out"=w324:errorcluster, "Array"=w330:string[][])  [unwired: 7 in]
            n148 = Number To Decimal String(number=w346) -> (decimal integer string=w343:string[])  [unwired: 1 in]
            n149 = Index Array(array=w330) -> (element=w329:string[])  [unwired: 2 in]
            n150 = Index Array(array=w329) -> (element=w328:string)  [unwired: 1 in]
            n151 = property class="MCListbox (严格)"(reference=w345, error in=w324, "RowHdrs[]"=w343, "ItemNames"=w342, "TopLeft"=w344) -> (error out=w323:errorcluster)  [unwired: 1 out]
            n152 = One Button Dialog(message=w328) -> ()  [unwired: 1 in, 1 out]
          }
        }
        n153 = property class="Bool (严格)"(reference=w320, error in=w314, "Value"=FALSE ("值")) -> (error out=w312:errorcluster)  [unwired: 1 out]
      }
      event "产品条码": Value Change {
        n154 = event-data() -> ("NewVal"=w367:string)  [unwired: 1 in]
        n155 = global read "GlobalV.vi" "SelfMode"() -> (w391:string[])
        n156 = property class="Ring (严格)"(reference=w378, error in=w371) -> (error out=w392:errorcluster, "RingText.Text"=w366:string)  [unwired: 1 out]
        n157 = property class="Str"(reference=w381, "DisabledEnum"=2) -> (reference out=w379:refnum<vi>)  [unwired: 1 in, 1 out]
        n158 = Index Array(array=w391, index #1=0 ("索引"), index #2=1 ("索引"), index #3=2 ("索引")) -> (element #1=w374:string, element #2=w373:string, element #3=w377:string)
        n159 = String Length(string=w373) -> (length=w386:i32)
        n160 = String Length(string=w367) -> (length=w375:i32)
        n161 = Decimal String To Number(string=w374) -> (number=w387:i32)  [unwired: 2 in, 1 out]
        n162 = String Subset(string=w367, length (rest)=w386) -> (substring=w385:string)  [unwired: 1 in]
        n163 = call "ModelCovert.vi"("ModelIn"=w366) -> ("ModelOut"=w365:string)  [unwired: 9 in, 1 out]
        n164 = Equal?(x=w375, y=w387) -> (x = y?=w384:bool)
        n165 = Equal?(x=w385, y=w373) -> (x = y?=w383:bool)
        n166 = And(x=w384, y=w383) -> (x .and. y?=w382:bool)
        n167 = case shown="真" w382 {
          tunnel: w365 -> [_ w427]
          tunnel: w392 -> [w403 w423]
          tunnel: [w395 w422] -> w370
          tunnel: w367 -> [_ w421]
          tunnel: w379 -> [w398 w420]
          tunnel: w377 -> [_ w419]
          tunnel: w376 -> [_ w418]
          tunnel: w375 -> [w402 _]
          tunnel: w374 -> [w401 _]
          tunnel: w373 -> [w400 _]
          tunnel: w372 -> [_ w417]
          frame False {
            n168 = flat-sequence {
              tunnel: [w410] -> w404
              tunnel: w403 -> [w410]
              tunnel: w402 -> [w409]
              tunnel: w401 -> [w408]
              tunnel: w400 -> [w407]
              tunnel: [w406] -> w399
              tunnel: w398 -> [w406]
              frame #0 {
                n169 = Number To Decimal String(number=w409) -> (decimal integer string=w414:string)  [unwired: 1 in]
                n170 = Concatenate Strings("条码长度或前置规则不匹配，请检查后重试！\n" ("消息"), "实际条码长度 ", w414, "，要求条码长度 ", w408, "\n前置规则要求：" ("字符串"), w407) -> (w412:string)
                n171 = One Button Dialog(message=w412) -> ()  [unwired: 1 in, 1 out]
              }
            }
            n172 = property class="Str"(reference=w399, error in=w404, "Value"="", "DisabledEnum"=0) -> (reference out=w394:refnum<vi>, error out=w396:errorcluster)
            n173 = property class="Str"(reference=w394, error in=w396, "Key Focus"=TRUE) -> (error out=w395:errorcluster)  [unwired: 1 out]
          }
          frame True {
            n174 = Concatenate Strings("'" ("字符串"), w427, "','" ("字符串"), w421, "',@A" ("字符串")) -> (w429:string)
            n175 = call "DBGetData.vi"("String"=w429, "Procedure"="prc_PackGetdata") -> ("Data Out"=w428:string[][])  [unwired: 8 in, 1 out]
            n176 = Index Array(array=w428) -> (element=w425:string[])  [unwired: 2 in]
            n177 = Array Size(array=w425) -> (size(s)=w426:i32)
            n178 = case shown="1" w426 {
              tunnel: w425 -> [_ w455 w487]
              tunnel: w423 -> [w436 w454 w479]
              tunnel: [w435 w449 w475] -> w422
              tunnel: w420 -> [w433 w451 w474]
              tunnel: w419 -> [_ _ w472]
              tunnel: w418 -> [_ _ w470]
              tunnel: w417 -> [_ _ w469]
              frame -1, 0, Default {
                n179 = flat-sequence {
                  tunnel: [w439] -> w437
                  tunnel: w436 -> [w439]
                  tunnel: [w438] -> w434
                  tunnel: w433 -> [w438]
                  tunnel: w437 -> [w443]
                  tunnel: [w442] -> w435
                  tunnel: w434 -> [w441]
                  frame #0 {
                    n180 = One Button Dialog(message="您输入的SN未通过测试！\n或\n外部条码与内部条码不一致，请检查！" ("消息")) -> ()  [unwired: 1 in, 1 out]
                  }
                  frame #1 {
                    n181 = property class="Str"(reference=w441, error in=w443, "Key Focus"=TRUE ("键选中"), "Value"="", "DisabledEnum"=T3."Enabled" ("禁用")) -> (error out=w442:errorcluster)  [unwired: 1 out]
                  }
                }
              }
              frame 1 {
                n182 = flat-sequence {
                  tunnel: w455 -> [w459]
                  tunnel: w454 -> [w457]
                  tunnel: [w457] -> w453
                  tunnel: [w456] -> w452
                  tunnel: w451 -> [w456]
                  tunnel: w453 -> [w463]
                  tunnel: [w462] -> w450
                  tunnel: w452 -> [w461]
                  tunnel: [w460] -> w448
                  frame #0 {
                    n183 = Index Array(array=w459) -> (element=w458:string)  [unwired: 1 in]
                    n184 = One Button Dialog(message=w458) -> ()  [unwired: 1 in, 1 out]
                  }
                  frame #1 {
                    n185 = property class="Str"(reference=w461, error in=w463, "Key Focus"=TRUE ("键选中"), "Value"="", "DisabledEnum"=T3."Enabled" ("禁用")) -> (reference out=w460:refnum<vi>, error out=w462:errorcluster)
                  }
                }
                n186 = property class="Str"(reference=w448, error in=w450, "Key Focus"=TRUE ("键选中")) -> (error out=w449:errorcluster)  [unwired: 1 out]
              }
              frame 2..8 {
                n187 = flat-sequence {
                  tunnel: w487 -> [w511]
                  tunnel: [w509] -> w486
                  tunnel: [w508] -> w485
                  tunnel: [w507] -> w482
                  tunnel: [w506] -> w484
                  tunnel: [w503] -> w481
                  tunnel: w479 -> [w502]
                  tunnel: [w501] -> w478
                  tunnel: [w500] -> w473
                  tunnel: w474 -> [w500]
                  tunnel: w472 -> [w499]
                  tunnel: [w498] -> w471
                  tunnel: w470 -> [w498]
                  tunnel: w469 -> [w497]
                  frame #0 {
                    n188 = property class="MCListbox (严格)"(reference=w497, error in=w502) -> (reference out=w509:refnum<vi>, error out=w501:errorcluster, "ItemNames"=w512:string[][])
                    n189 = Decimal String To Number(string=w499) -> (number=w504:i32)  [unwired: 2 in, 1 out]
                    n190 = Array Size(array=w512) -> (size(s)=w513:i32[])
                    n191 = Insert Into Array(array=w512, new element=w511) -> (w506:string[][])  [unwired: 2 in]
                    n192 = Index Array(array=w513) -> (element=w514:i32)  [unwired: 1 in]
                    n193 = Increment(x=w514) -> (x+1=w505:i32)
                    n194 = for {
                      N: w505 -> [_]
                      tunnel: [w515] -> w510 mode=indexing
                      tunnel: [w516] -> w507
                      i -> [w516]
                      n195 = Increment(x=w516) -> (x+1=w515:i32)
                    }
                    n196 = Greater Or Equal?(x=w505, y=w504) -> (x >= y?=w503:bool)
                    n197 = Number To Decimal String(number=w510) -> (decimal integer string=w508:string[])  [unwired: 1 in]
                  }
                }
                n198 = call "TopLeft position.vi"("index"=w482) -> ("TopLeft"=w483:T4)
                n199 = property class="MCListbox (严格)"(reference=w486, error in=w478, "RowHdrs[]"=w485, "Value"=w482, "ItemNames"=w484, "TopLeft"=w483) -> (error out=w477:errorcluster)  [unwired: 1 out]
                n200 = property class="Str"(reference=w473, error in=w477, "Value"="", "DisabledEnum"=0) -> (reference out=w480:refnum<vi>, error out=w476:errorcluster)
                n201 = case shown="真" w481 {
                  tunnel: w480 -> [w489 w492]
                  tunnel: w476 -> [w490 w495]
                  tunnel: [w490 w494] -> w475
                  tunnel: w471 -> [_ w493]
                  frame False {
                    n202 = property class="Str"(reference=w489, "Key Focus"=TRUE) -> ()  [unwired: 1 in, 2 out]
                  }
                  frame True {
                    n203 = property class="Str"(reference=w492, "Key Focus"=TRUE) -> ()  [unwired: 1 in, 2 out]
                    n204 = Generate User Event(user event=w493, event data cluster="WriteDataToDB" ("事件数据"), error in=w495) -> (error out=w494:errorcluster)  [unwired: 1 in, 1 out]
                  }
                }
              }
            }
          }
        }
      }
      event User Event {
        n205 = event-data() -> ("SelfPack"=w527:string)  [unwired: 1 in]
        n206 = property class="Ring (严格)"(reference=w525) -> ("RingText.Text"=w524:string)  [unwired: 1 in, 2 out]
        n207 = Unbundle By Name(w518) -> ("料号"=w517:refnum<vi>)
        n208 = case shown="\"WriteDataToDB\"" w527 {
          tunnel: w526 -> [_ w569]
          tunnel: w524 -> [_ w536]
          tunnel: w523 -> [_ w545]
          tunnel: w522 -> [w528 w540]
          tunnel: [w528 w538] -> w521
          tunnel: w517 -> [_ w533]
          frame "假", Default {
          }
          frame "WriteDataToDB" {
            w561 = "'"
            w560 = ","
            n209 = property class="Str"(reference=w533) -> ("Value"=w530:string)  [unwired: 1 in, 2 out]
            n210 = property class="MCListbox (严格)"(reference=w569, error in=w540) -> (reference out=w553:refnum<vi>, error out=w539:errorcluster, "ItemNames"=w542:string[][])
            n211 = property class="Str"(reference=w545) -> ("Value"=w535:string)  [unwired: 1 in, 2 out]
            n212 = call "ModelCovert.vi"("ModelIn"=w536) -> ("ModelOut"=w537:string)  [unwired: 9 in, 1 out]
            n213 = Format Date/Time String(time format string (%c)="%Y%m%d" ("时间格式字符串(%c)")) -> (date/time string=w549:string)  [unwired: 2 in]
            n214 = String Subset(string=w549, offset (0)=2 ("偏移量(0)")) -> (substring=w547:string)  [unwired: 1 in]
            n215 = for {
              tunnel: w542 -> [w603] mode=indexing
              shift-right: [w600] -> w565
              shift-left: "" -> [w602]
              n216 = Index Array(array=w603, index=2 ("索引")) -> (element=w601:string)
              n217 = Concatenate Strings(w602, w601, ",") -> (w600:string)
            }
            n218 = Concatenate Strings("地址：", w535, "\n", "料号：", w530) -> (w529:string)
            n219 = call "GetBoxNo.vi"("error in"=w539, "种类"=enum16{"自产", "外购"}."自产", "TimeStr"=w547, "Model"=w537) -> ("error out"=w543:errorcluster, "BoxNo"=w546:string)  [unwired: 6 in]
            n220 = Format Date/Time String(time format string (%c)="%Y-%m-%d %H:%M:%S" ("时间格式字符串(%c)")) -> (date/time string=w562:string)  [unwired: 2 in]
            n221 = String Length(string=w565) -> (length=w567:i32)
            n222 = Decrement(x=w567) -> (x-1=w566:i32)
            n223 = String Subset(string=w565, length (rest)=w566) -> (substring=w563:string)  [unwired: 1 in]
            n224 = Concatenate Strings(w561, w537, w561, w560, w561, w546, w561, w560, w561, w563, w561, w560, w561, w535, w561, w560, w561, w562, w561, w560, "@A" ("字符串")) -> (w558:string)
            n225 = call "prc_writeBOXdata.vi"("error in"=w543, "string"=w558, "Process"="prc_MPackForPrint") -> ("error out"=w541:errorcluster, "Array"=w557:string[][])  [unwired: 7 in]
            n226 = Index Array(array=w557) -> (element=w556:string[])  [unwired: 2 in]
            n227 = Index Array(array=w556) -> (element=w552:string)  [unwired: 1 in]
            n228 = Equal?(x=w552, y="OK") -> (x = y?=w554:bool)
            n229 = case shown="真" w554 {
              tunnel: w553 -> [_ w597]
              tunnel: w552 -> [w571 _]
              tunnel: w542 -> [_ w578]
              tunnel: w536 -> [_ w575]
              tunnel: w541 -> [w570 w577]
              tunnel: [w570 w580] -> w538
              tunnel: w529 -> [_ w573]
              frame False {
                n230 = One Button Dialog(message=w571) -> ()  [unwired: 1 in, 1 out]
              }
              frame True {
                w574 = 2 ("Index")
                n231 = call "TxtFlash.vi"("Index"=w574, "Adress"=w573, "error in"=w577, "Model"=w575, "ItemNames"=w578, "Path"="Config\\MidBox\\Adress.txt") -> ("error out"=w576:errorcluster)  [unwired: 5 in]
                n232 = call "TxtFlash.vi"("Index"=w574, "error in"=w577, "Model"=w575, "ItemNames"=w578, "Path"="Config\\MidBox\\Date.txt") -> ("error out"=w589:errorcluster)  [unwired: 6 in]
                n233 = call "TxtFlash.vi"("Index"=w574, "error in"=w577, "Model"=w575, "ItemNames"=w578, "Path"="Config\\MidBox\\Number.txt") -> ("error out"=w590:errorcluster)  [unwired: 6 in]
                n234 = call "TxtFlash.vi"("Index"=w574, "error in"=w577, "Model"=w575, "ItemNames"=w578, "Path"="Config\\MidBox\\SN.txt") -> ("error out"=w591:errorcluster)  [unwired: 6 in]
                n235 = call "TxtFlash.vi"("Index"=w574, "error in"=w577, "Model"=w575, "ItemNames"=w578, "Path"="Config\\MidBox\\Model.txt") -> ("error out"=w592:errorcluster)  [unwired: 6 in]
                n236 = Merge Errors(w576, w589, w590, w591, w592) -> (w572:errorcluster)
                n237 = invoke class="MCListbox (严格)" method="Reinit To Default"(reference=w597, error in=w572) -> (reference out=w596:refnum<vi>, error out=w583:errorcluster)  [unwired: 1 in, 1 out]
                n238 = property class="MCListbox (严格)"(reference=w596, error in=w583, "SelColor"=u32 16775631, "RowHdrs[]"=string[] [] ("行首字符串[]"), "ItemNames"=string[][] [] ("项名")) -> (error out=w581:errorcluster)  [unwired: 1 out]
                n239 = call "StickerPrint.vi"("error in"=w572, "Path"="Config\\MidBox\\58102.btw") -> ("error out"=w582:errorcluster)  [unwired: 9 in]
                n240 = Merge Errors(w581, w582) -> (w580:errorcluster)
              }
            }
          }
        }
      }
      event Menu Selection (User) {
        n241 = event-data() -> ("ItemTag"=w607:string)  [unwired: 1 in]
        n242 = case shown="\"Bprint\"" w607 {
          tunnel: w606 -> [_ w611 w630 w651 w671 w690 w700 w717 w734]
          frame "假", Default {
          }
          frame "SelfPack" {
            n243 = Unbundle By Name(w611) -> ("选项"=w610:refnum<vi>)
            n244 = call "Login.vi"("ps"="123456", "User"="Sroot") -> ("Access"=w612:bool)  [unwired: 9 in]
            n245 = case shown="真" w612 {
              tunnel: w610 -> [w616 w622]
              tunnel: enum32{"自产包装", "外购机BSJ包装", "出货", "大箱条码打印"}."自产包装" ("值") -> [_ w621]
              frame False {
                n246 = property class="TabCtl (严格)"(reference=w616) -> ("Pages"=w615:refnum<vi>[])  [unwired: 1 in, 2 out]
                n247 = for {
                  tunnel: w615 -> [w618] mode=indexing
                  n248 = property class="Page"(reference=w618, "PageEnb"=2) -> ()  [unwired: 1 in, 2 out]
                }
              }
              frame True {
                w619 = 2
                n249 = property class="TabCtl (严格)"(reference=w622) -> ("Pages"=w627:refnum<vi>[])  [unwired: 1 in, 2 out]
                n250 = property class="TabCtl (严格)"(reference=w622, "Value"=w621) -> ()  [unwired: 1 in, 2 out]
                n251 = Index Array(array=w627) -> (element #1=w626:refnum<vi>, element #2=w625:refnum<vi>, element #3=w624:refnum<vi>, element #4=w620:refnum<vi>)  [unwired: 4 in]
                n252 = property class="Page"(reference=w626, "PageEnb"=0) -> ()  [unwired: 1 in, 2 out]
                n253 = property class="Page"(reference=w625, "PageEnb"=w619) -> ()  [unwired: 1 in, 2 out]
                n254 = property class="Page"(reference=w624, "PageEnb"=w619) -> ()  [unwired: 1 in, 2 out]
                n255 = property class="Page"(reference=w620, "PageEnb"=w619) -> ()  [unwired: 1 in, 2 out]
              }
            }
          }
          frame "InPack" {
            n256 = Unbundle By Name(w630) -> ("选项"=w629:refnum<vi>)
            n257 = call "Login.vi"("ps"="123456", "User"="Iroot") -> ("Access"=w631:bool)  [unwired: 9 in]
            n258 = case shown="假" w631 {
              tunnel: w629 -> [w635 w641]
              tunnel: enum32{"自产包装", "外购机BSJ包装", "出货", "大箱条码打印"}."外购机BSJ包装" ("值") -> [_ w640]
              frame False {
                n259 = property class="TabCtl (严格)"(reference=w635) -> ("Pages"=w634:refnum<vi>[])  [unwired: 1 in, 2 out]
                n260 = for {
                  tunnel: w634 -> [w637] mode=indexing
                  n261 = property class="Page"(reference=w637, "PageEnb"=2) -> ()  [unwired: 1 in, 2 out]
                }
              }
              frame True {
                n262 = property class="TabCtl (严格)"(reference=w641, "Value"=w640) -> ()  [unwired: 1 in, 2 out]
                n263 = property class="TabCtl (严格)"(reference=w641) -> ("Pages"=w648:refnum<vi>[])  [unwired: 1 in, 2 out]
                n264 = Index Array(array=w648) -> (element #1=w647:refnum<vi>, element #2=w646:refnum<vi>, element #3=w645:refnum<vi>, element #4=w638:refnum<vi>)  [unwired: 4 in]
                n265 = property class="Page"(reference=w647, "PageEnb"=2) -> ()  [unwired: 1 in, 2 out]
                n266 = property class="Page"(reference=w646, "PageEnb"=0) -> ()  [unwired: 1 in, 2 out]
                n267 = property class="Page"(reference=w645, "PageEnb"=2) -> ()  [unwired: 1 in, 2 out]
                n268 = property class="Page"(reference=w638, "PageEnb"=2) -> ()  [unwired: 1 in, 2 out]
              }
            }
          }
          frame "Export" {
            n269 = Unbundle By Name(w651) -> ("选项"=w650:refnum<vi>)
            n270 = call "Login.vi"("ps"="123456", "User"="Eroot") -> ("Access"=w652:bool)  [unwired: 9 in]
            n271 = case shown="真" w652 {
              tunnel: w650 -> [w655 w662]
              tunnel: enum32{"自产包装", "外购机BSJ包装", "出货", "大箱条码打印"}."出货" ("值") -> [_ w661]
              frame False {
                n272 = property class="TabCtl (严格)"(reference=w655) -> ("Pages"=w656:refnum<vi>[])  [unwired: 1 in, 2 out]
                n273 = for {
                  tunnel: w656 -> [w658] mode=indexing
                  n274 = property class="Page"(reference=w658, "PageEnb"=2) -> ()  [unwired: 1 in, 2 out]
                }
              }
              frame True {
                w660 = 2
                n275 = property class="TabCtl (严格)"(reference=w662, "Value"=w661) -> ()  [unwired: 1 in, 2 out]
                n276 = property class="TabCtl (严格)"(reference=w662) -> ("Pages"=w668:refnum<vi>[])  [unwired: 1 in, 2 out]
                n277 = Index Array(array=w668) -> (element #1=w667:refnum<vi>, element #2=w666:refnum<vi>, element #3=w665:refnum<vi>, element #4=w659:refnum<vi>)  [unwired: 4 in]
                n278 = property class="Page"(reference=w667, "PageEnb"=2) -> ()  [unwired: 1 in, 2 out]
                n279 = property class="Page"(reference=w666, "PageEnb"=w660) -> ()  [unwired: 1 in, 2 out]
                n280 = property class="Page"(reference=w665, "PageEnb"=0) -> ()  [unwired: 1 in, 2 out]
                n281 = property class="Page"(reference=w659, "PageEnb"=w660) -> ()  [unwired: 1 in, 2 out]
              }
            }
          }
          frame "BigPack" {
            n282 = Unbundle By Name(w671) -> ("选项"=w670:refnum<vi>)
            n283 = call "Login.vi"("ps"="123456", "User"="Broot") -> ("Access"=w672:bool)  [unwired: 9 in]
            n284 = case shown="假" w672 {
              tunnel: w670 -> [w675 w681]
              tunnel: enum32{"自产包装", "外购机BSJ包装", "出货", "大箱条码打印"}."大箱条码打印" ("值") -> [_ w683]
              frame False {
                n285 = property class="TabCtl (严格)"(reference=w675) -> ("Pages"=w676:refnum<vi>[])  [unwired: 1 in, 2 out]
                n286 = for {
                  tunnel: w676 -> [w678] mode=indexing
                  n287 = property class="Page"(reference=w678, "PageEnb"=2) -> ()  [unwired: 1 in, 2 out]
                }
              }
              frame True {
                w679 = 2
                n288 = property class="TabCtl (严格)"(reference=w681, "Value"=w683) -> ()  [unwired: 1 in, 2 out]
                n289 = property class="TabCtl (严格)"(reference=w681) -> ("Pages"=w688:refnum<vi>[])  [unwired: 1 in, 2 out]
                n290 = Index Array(array=w688) -> (element #1=w682:refnum<vi>, element #2=w687:refnum<vi>, element #3=w686:refnum<vi>, element #4=w684:refnum<vi>)  [unwired: 4 in]
                n291 = property class="Page"(reference=w682, "PageEnb"=2) -> ()  [unwired: 1 in, 2 out]
                n292 = property class="Page"(reference=w687, "PageEnb"=w679) -> ()  [unwired: 1 in, 2 out]
                n293 = property class="Page"(reference=w686, "PageEnb"=w679) -> ()  [unwired: 1 in, 2 out]
                n294 = property class="Page"(reference=w684, "PageEnb"=0) -> ()  [unwired: 1 in, 2 out]
              }
            }
          }
          frame "FlashModel" {
            n295 = Unbundle By Name(w690) -> ("选项"=w689:refnum<vi>)
            n296 = call "Login.vi"("ps"="123456", "User"="Froot") -> ("Access"=w691:bool)  [unwired: 9 in]
            n297 = case shown="真" w691 {
              tunnel: w689 -> [w694 _]
              frame False {
                n298 = property class="TabCtl (严格)"(reference=w694) -> ("Pages"=w695:refnum<vi>[])  [unwired: 1 in, 2 out]
                n299 = for {
                  tunnel: w695 -> [w697] mode=indexing
                  n300 = property class="Page"(reference=w697, "PageEnb"=2) -> ()  [unwired: 1 in, 2 out]
                }
              }
              frame True {
                n301 = call "FlashModel.vi"() -> ()  [unwired: 12 in]
              }
            }
          }
          frame "Logout" {
            n302 = Unbundle By Name(w700) -> ("选项"=w699:refnum<vi>)
            n303 = disable-structure shown="启用" {
              disable-tunnel: [w702 TRUE] -> w701
              frame Disabled {
                n304 = call "Login.vi"("ps"="123456", "User"="Lroot") -> ("Access"=w702:bool)  [unwired: 9 in]
              }
              frame Enabled {
              }
            }
            n305 = case shown="真" w701 {
              tunnel: w699 -> [w706 w712]
              tunnel: enum32{"自产包装", "外购机BSJ包装", "出货", "大箱条码打印"}."自产包装" ("值") -> [_ w710]
              frame False {
                n306 = property class="TabCtl (严格)"(reference=w706) -> ("Pages"=w707:refnum<vi>[])  [unwired: 1 in, 2 out]
                n307 = for {
                  tunnel: w707 -> [w709] mode=indexing
                  n308 = property class="Page"(reference=w709, "PageEnb"=2) -> ()  [unwired: 1 in, 2 out]
                }
              }
              frame True {
                n309 = property class="TabCtl (严格)"(reference=w712, "Value"=w710) -> ()  [unwired: 1 in, 2 out]
                n310 = property class="TabCtl (严格)"(reference=w712) -> ("Pages"=w711:refnum<vi>[])  [unwired: 1 in, 2 out]
                n311 = for {
                  tunnel: w711 -> [w714] mode=indexing
                  n312 = property class="Page"(reference=w714, "PageEnb"=2) -> ()  [unwired: 1 in, 2 out]
                }
              }
            }
          }
          frame "Bprint" {
            n313 = Unbundle By Name(w717) -> ("选项"=w716:refnum<vi>)
            n314 = disable-structure shown="启用" {
              disable-tunnel: [w719 TRUE] -> w718
              frame Enabled {
                n315 = call "Login.vi"("ps"="123456", "User"="MProot") -> ("Access"=w719:bool)  [unwired: 9 in]
              }
              frame Disabled {
              }
            }
            n316 = case shown="真" w718 {
              tunnel: w716 -> [w723 w730]
              tunnel: enum32{"自产包装", "外购机BSJ包装", "出货", "大箱条码打印"}."自产包装" ("值") -> [_ w731]
              frame False {
                n317 = disable-structure shown="禁用" {
                  disable-tunnel: w723 -> [w724 _]
                  frame Disabled {
                    n318 = property class="TabCtl (严格)"(reference=w724) -> ("Pages"=w725:refnum<vi>[])  [unwired: 1 in, 2 out]
                    n319 = for {
                      tunnel: w725 -> [w727] mode=indexing
                      n320 = property class="Page"(reference=w727, "PageEnb"=2) -> ()  [unwired: 1 in, 2 out]
                    }
                  }
                  frame Enabled {
                  }
                }
              }
              frame True {
                n321 = property class="TabCtl (严格)"(reference=w730, "Value"=w731) -> (error out=w728:errorcluster)  [unwired: 1 in, 1 out]
                n322 = call "StickerPrint.vi"("error in"=w728, "Path"="Config\\MidBox\\58102.btw") -> ()  [unwired: 9 in, 1 out]
              }
            }
          }
          frame "BigPrint" {
            n323 = Unbundle By Name(w734) -> ("选项"=w733:refnum<vi>)
            n324 = disable-structure shown="启用" {
              disable-tunnel: [w736 TRUE] -> w735
              frame Enabled {
                n325 = call "Login.vi"("ps"="123456", "User"="BProot") -> ("Access"=w736:bool)  [unwired: 9 in]
              }
              frame Disabled {
              }
            }
            n326 = case shown="真" w735 {
              tunnel: w733 -> [w740 w747]
              tunnel: enum32{"自产包装", "外购机BSJ包装", "出货", "大箱条码打印"}."大箱条码打印" ("值") -> [_ w748]
              frame False {
                n327 = disable-structure shown="启用" {
                  disable-tunnel: w740 -> [w741 _]
                  frame Disabled {
                    n328 = property class="TabCtl (严格)"(reference=w741) -> ("Pages"=w742:refnum<vi>[])  [unwired: 1 in, 2 out]
                    n329 = for {
                      tunnel: w742 -> [w744] mode=indexing
                      n330 = property class="Page"(reference=w744, "PageEnb"=2) -> ()  [unwired: 1 in, 2 out]
                    }
                  }
                  frame Enabled {
                  }
                }
              }
              frame True {
                n331 = property class="TabCtl (严格)"(reference=w747, "Value"=w748) -> (error out=w746:errorcluster)  [unwired: 1 in, 1 out]
                n332 = call "StickerPrint.vi"("error in"=w746, "Path"="Config\\BigBox\\102152.btw") -> ()  [unwired: 9 in, 1 out]
              }
            }
          }
        }
      }
      event "设定大箱总数": Value Change {
        n333 = event-data() -> ("CtlRef"=w755:refnum<vi>, "NewVal"=w754:i32)  [unwired: 1 in]
        n334 = Greater Or Equal To 0?(x=w754) -> (x >= 0?=w756:bool)
        n335 = To Unsigned Long Integer(number=w754) -> (unsigned 32bit integer=w753:u32)
        n336 = case shown="假" w756 {
          tunnel: w755 -> [w760 w768]
          tunnel: w752 -> [w758 w765]
          tunnel: [w757 w764] -> w751
          tunnel: w753 -> [_ w762]
          frame False {
            n337 = property class="DigNum (严格)"(reference=w760, error in=w758, "DisabledEnum"=0) -> (error out=w757:errorcluster)  [unwired: 1 out]
            n338 = One Button Dialog(message="出货数量为0，请设置正确的出货数量！" ("消息")) -> ()  [unwired: 1 in, 1 out]
          }
          frame True {
            n339 = flat-sequence {
              tunnel: [w774] -> w769
              tunnel: w768 -> [w773]
              tunnel: [w773] -> w767
              tunnel: [w772] -> w766
              tunnel: w765 -> [w772]
              tunnel: [w771] -> w763
              tunnel: w762 -> [w771]
              tunnel: w769 -> [w781]
              tunnel: w767 -> [w780]
              tunnel: w766 -> [w779]
              tunnel: [w778] -> w764
              tunnel: w763 -> [w777]
              frame #0 {
                n340 = Number To Decimal String(number=w771) -> (decimal integer string=w770:string)  [unwired: 1 in]
                n341 = Concatenate Strings("本次出货数量为：" ("消息"), w770) -> (w775:string)
                n342 = Two Button Dialog(message=w775) -> (T button?=w774:bool)  [unwired: 2 in]
              }
              frame #1 {
                n343 = case shown="真" w781 {
                  tunnel: w780 -> [w786 w792]
                  tunnel: w779 -> [w784 w790]
                  tunnel: [w783 w789] -> w778
                  tunnel: w777 -> [_ w788]
                  frame False {
                    n344 = property class="DigNum (严格)"(reference=w786, error in=w784, "DisabledEnum"=0, "Key Focus"=TRUE, "Value"=0) -> (error out=w783:errorcluster)  [unwired: 1 out]
                  }
                  frame True {
                    n345 = property class="DigNum (严格)"(reference=w792, error in=w790, "DisabledEnum"=2, "Value"=w788) -> (error out=w789:errorcluster)  [unwired: 1 out]
                  }
                }
              }
            }
          }
        }
      }
      event "手动计数打印？": Value Change {
        n346 = event-data() -> ("NewVal"=w798:bool)  [unwired: 1 in]
        n347 = Unbundle By Name(w799) -> ("手动打印"=w797:refnum<vi>)
        n348 = property class="Bool (严格)"(reference=w797, error in=w796, "Visible"=w798) -> (error out=w795:errorcluster)  [unwired: 1 out]
      }
      event "条码": Value Change {
        n349 = event-data() -> ("CtlRef"=w818:refnum<vi>, "NewVal"=w821:string)  [unwired: 1 in]
        n350 = property class="DigNum (严格)"(reference=w810) -> (reference out=w809:refnum<vi>, "Value"=w812:i32)  [unwired: 1 in, 1 out]
        n351 = Unbundle By Name(w817) -> ("大箱内产品"=w816:refnum<vi>, "类别"=w804:refnum<vi>)
        n352 = Empty String/Path?(string/path=w821) -> (empty?=w814:bool)
        n353 = property class="Ring (严格)"(reference=w804) -> ("RingText.Text"=w803:string)  [unwired: 1 in, 2 out]
        n354 = Less Or Equal To 0?(x=w812) -> (x <= 0?=w815:bool)
        n355 = Or(x=w814, y=w815) -> (x .or. y?=w813:bool)
        n356 = Equal?(x=w803, y="外购") -> (x = y?=w801:bool)
        n357 = case shown="假" w813 {
          tunnel: w821 -> [w838 _]
          tunnel: w820 -> [w833 w999]
          tunnel: [w835 w999] -> w819
          tunnel: w818 -> [w842 w994]
          tunnel: w816 -> [w841 _]
          tunnel: w800 -> [w839 w998]
          tunnel: w812 -> [w832 _]
          tunnel: w811 -> [w837 _]
          tunnel: w809 -> [w836 _]
          tunnel: w808 -> [w834 _]
          tunnel: [w831 w998] -> w807
          tunnel: [w830 w993] -> w806
          tunnel: w805 -> [w829 w997]
          tunnel: w801 -> [w828 _]
          tunnel: w800 -> [w825 _]
          frame False {
            n358 = call "BreakStr.vi"("error in"=w829, "外购？"=w828, "StrIn"=w838) -> ("error out"=w824:errorcluster, "ArrayOut"=w826:string[])  [unwired: 7 in]
            n359 = call "MidBoxScanRepeatCheck.vi"("error in"=w824, "StrIn"=w825, "ArrayIn"=w826) -> ("error out"=w823:errorcluster, "StrOut"=w822:string, "OK？"=w827:bool)  [unwired: 6 in]
            n360 = case shown="真" w827 {
              tunnel: w842 -> [w846 w885]
              tunnel: w841 -> [_ w884]
              tunnel: 2 -> [_ w883]
              tunnel: w839 -> [w849 w881]
              tunnel: w837 -> [_ w877]
              tunnel: w836 -> [_ w875]
              tunnel: [w848 w874] -> w835
              tunnel: w834 -> [_ w873]
              tunnel: w833 -> [w848 w872]
              tunnel: w832 -> [_ w870]
              tunnel: [w849 w869] -> w831
              tunnel: [w843 w868] -> w830
              tunnel: w823 -> [w847 w867]
              tunnel: w826 -> [_ w866]
              tunnel: w822 -> [w850 _]
              frame False {
                n361 = flat-sequence {
                  tunnel: w850 -> [w854]
                  tunnel: w847 -> [w851]
                  tunnel: w846 -> [w852]
                  tunnel: [w852] -> w845
                  tunnel: [w851] -> w844
                  tunnel: w845 -> [w863]
                  tunnel: w844 -> [w858]
                  tunnel: [w857] -> w843
                  frame #0 {
                    n362 = Concatenate Strings("部分产品已重扫！" ("字符串"), "\n", w854) -> (w853:string)
                    n363 = One Button Dialog(message=w853) -> ()  [unwired: 1 in, 1 out]
                  }
                  frame #1 {
                    n364 = property class="Str"(reference=w863, error in=w858, "DisabledEnum"=0, "Value"="") -> (reference out=w861:refnum<vi>, error out=w859:errorcluster)
                    n365 = property class="Str"(reference=w861, error in=w859, "Key Focus"=TRUE) -> (error out=w857:errorcluster)  [unwired: 1 out]
                  }
                }
              }
              frame True {
                n366 = Array Size(array=w866) -> (size(s)=w882:i32)
                n367 = call "ArrayToStr.vi"("Array"=w866) -> ("Str"=w865:string)
                n368 = property class="Str"(reference=w885, error in=w867, "DisabledEnum"=w883) -> (reference out=w878:refnum<vi>, error out=w876:errorcluster)
                n369 = To Unsigned Long Integer(number=w882) -> (unsigned 32bit integer=w879:u32)
                n370 = Add(x=w872, y=w879) -> (x+y=w871:u32)
                n371 = Greater?(x=w871, y=w870) -> (0:w880:bool)
                n372 = case shown="真" w880 {
                  tunnel: w884 -> [w893 w962]
                  tunnel: w881 -> [w895 w947]
                  tunnel: w865 -> [w894 w961]
                  tunnel: w872 -> [_ w959]
                  tunnel: w879 -> [_ w955]
                  tunnel: w878 -> [w892 w949]
                  tunnel: w877 -> [w891 w948]
                  tunnel: w876 -> [w896 w944]
                  tunnel: w875 -> [_ _]
                  tunnel: w871 -> [_ w943]
                  tunnel: [w888 w942] -> w874
                  tunnel: w873 -> [w889 w941]
                  tunnel: w872 -> [_ w940]
                  tunnel: w871 -> [w890 _]
                  tunnel: w870 -> [w898 _]
                  tunnel: [w887 w939] -> w869
                  tunnel: [w886 w938] -> w868
                  frame False {
                    n373 = Equal?(x=w890, y=w898) -> (x = y?=w897:bool)
                    n374 = case shown="假" w897 {
                      tunnel: w896 -> [w915 w934]
                      tunnel: w895 -> [w913 w932]
                      tunnel: w894 -> [w911 w930]
                      tunnel: w893 -> [w910 w929]
                      tunnel: w892 -> [w907 w925]
                      tunnel: w891 -> [w906 _]
                      tunnel: w890 -> [w902 w922]
                      tunnel: w889 -> [w903 w923]
                      tunnel: [w902 w922] -> w888
                      tunnel: [w901 w920] -> w886
                      tunnel: [w899 w919] -> w887
                      frame True {
                        n375 = Empty String/Path?(string/path=w913) -> (empty?=w914:bool)
                        n376 = case shown="假" w914 {
                          tunnel: ["\n" ""] -> w912
                          frame False {
                          }
                          frame True {
                          }
                        }
                        n377 = Concatenate Strings(w913, w912, w911) -> (w899:string)
                        n378 = String Length(string=w899) -> (length=w916:i32)
                        n379 = property class="Str"(reference=w910, error in=w915, "Text.Text"=w899, "Text.Scroll Position"=w916) -> (error out=w900:errorcluster)  [unwired: 1 out]
                        n380 = property class="Str"(reference=w907, error in=w900, "DisabledEnum"=2, "Value"="") -> (error out=w904:errorcluster)  [unwired: 1 out]
                        n381 = Generate User Event(user event=w906, event data cluster="BarPrint", error in=w900) -> ()  [unwired: 1 in, 2 out]
                        n382 = property class="DigNum (严格)"(reference=w903, error in=w904, "Value"=w902) -> (error out=w901:errorcluster)  [unwired: 1 out]
                      }
                      frame False {
                        n383 = Empty String/Path?(string/path=w932) -> (empty?=w933:bool)
                        n384 = case shown="假" w933 {
                          tunnel: ["\n" ""] -> w931
                          frame False {
                          }
                          frame True {
                          }
                        }
                        n385 = Concatenate Strings(w932, w931, w930) -> (w919:string)
                        n386 = String Length(string=w919) -> (length=w935:i32)
                        n387 = property class="Str"(reference=w929, error in=w934, "Text.Text"=w919, "Text.Scroll Position"=w935) -> (error out=w927:errorcluster)  [unwired: 1 out]
                        n388 = property class="Str"(reference=w925, error in=w927, "DisabledEnum"=0, "Value"="", "Key Focus"=TRUE) -> (error out=w924:errorcluster)  [unwired: 1 out]
                        n389 = property class="DigNum (严格)"(reference=w923, error in=w924, "Value"=w922) -> (error out=w920:errorcluster)  [unwired: 1 out]
                      }
                    }
                  }
                  frame True {
                    w953 = "\n"
                    n390 = Number To Decimal String(number=w959) -> (decimal integer string=w957:string)  [unwired: 1 in]
                    n391 = Number To Decimal String(number=w955) -> (decimal integer string=w954:string)  [unwired: 1 in]
                    n392 = Empty String/Path?(string/path=w947) -> (empty?=w946:bool)
                    n393 = case shown="真" w946 {
                      tunnel: ["\n" ""] -> w945
                      frame False {
                      }
                      frame True {
                      }
                    }
                    n394 = Concatenate Strings("数量超过设定总数！" ("消息"), w953, "当前大箱内产品数：" ("消息"), w957, w953, "当前中箱内产品数：" ("消息"), w954, w953, "确定继续包装并打印条码？" ("消息")) -> (w951:string)
                    n395 = Two Button Dialog(message=w951) -> (T button?=w950:bool)  [unwired: 2 in]
                    n396 = case shown="真" w950 {
                      tunnel: w962 -> [_ w990]
                      tunnel: w947 -> [w973 w989]
                      tunnel: w961 -> [_ w988]
                      tunnel: w949 -> [w972 w982]
                      tunnel: w948 -> [_ w986]
                      tunnel: w945 -> [_ w984]
                      tunnel: w944 -> [w971 w983]
                      tunnel: w943 -> [_ w979]
                      tunnel: [w974 w979] -> w942
                      tunnel: w941 -> [_ w978]
                      tunnel: w940 -> [w974 _]
                      tunnel: [w973 w976] -> w939
                      tunnel: [w966 w975] -> w938
                      frame False {
                        n397 = property class="Str"(reference=w972, error in=w971, "DisabledEnum"=0, "Value"="") -> (reference out=w968:refnum<vi>, error out=w967:errorcluster)
                        n398 = property class="Str"(reference=w968, error in=w967, "Key Focus"=TRUE) -> (error out=w966:errorcluster)  [unwired: 1 out]
                      }
                      frame True {
                        n399 = Concatenate Strings(w989, w984, w988) -> (w976:string)
                        n400 = String Length(string=w976) -> (length=w987:i32)
                        n401 = property class="Str"(reference=w990, error in=w983, "Text.Text"=w976, "Text.Scroll Position"=w987) -> (error out=w977:errorcluster)  [unwired: 1 out]
                        n402 = property class="DigNum (严格)"(reference=w978, error in=w977, "Value"=w979) -> (error out=w975:errorcluster)  [unwired: 1 out]
                        n403 = Generate User Event(user event=w986, event data cluster="BarPrint", error in=w977) -> ()  [unwired: 1 in, 2 out]
                        n404 = property class="Str"(reference=w982, error in=w977, "DisabledEnum"=2, "Value"="") -> ()  [unwired: 2 out]
                      }
                    }
                  }
                }
              }
            }
          }
          frame True {
            n405 = flat-sequence {
              tunnel: [w1001] -> w996
              tunnel: w997 -> [w1001]
              tunnel: [w1000] -> w995
              tunnel: w994 -> [w1000]
              frame #0 {
                n406 = One Button Dialog(message="中箱条码内容为空或大箱总数设定值为0！请检查！" ("消息")) -> ()  [unwired: 1 in, 1 out]
              }
            }
            n407 = property class="Str"(reference=w995, error in=w996, "Value"="", "DisabledEnum"=0) -> (error out=w993:errorcluster)  [unwired: 1 out]
          }
        }
      }
      event "手动打印": Value Change {
        n408 = event-data() -> ("CtlRef"=w1005:refnum<vi>, "NewVal"=w1010:bool)  [unwired: 1 in]
        n409 = call "StrToArray.vi"("error in"=w1012, "StrIn"=w1011) -> ("error out"=w1009:errorcluster, "ArrayOut"=w1008:string[])  [unwired: 8 in]
        n410 = case shown="真" w1010 {
          tunnel: w1009 -> [w1014 w1019]
          tunnel: w1008 -> [_ w1024]
          tunnel: w1007 -> [_ w1020]
          tunnel: [w1014 w1018] -> w1006
          tunnel: w1005 -> [w1015 w1016]
          tunnel: [w1015 w1017] -> w1004
          frame False {
          }
          frame True {
            n411 = Array Size(array=w1024) -> (size(s)=w1023:i32)
            n412 = Greater Or Equal?(x=w1023, y=1) -> (x >= y?=w1021:bool)
            n413 = case shown="真" w1021 {
              tunnel: w1020 -> [_ w1032]
              tunnel: w1019 -> [w1026 w1030]
              tunnel: [w1026 w1029] -> w1018
              tunnel: [w1025 w1028] -> w1017
              tunnel: w1016 -> [w1025 w1028]
              frame False {
                n414 = One Button Dialog(message="包装箱数据为空！" ("消息")) -> ()  [unwired: 1 in, 1 out]
              }
              frame True {
                n415 = Generate User Event(user event=w1032, event data cluster="BarPrint", error in=w1030) -> (error out=w1029:errorcluster)  [unwired: 1 in, 1 out]
              }
            }
          }
        }
        n416 = property class="Bool (严格)"(reference=w1004, "Value"=FALSE ("值")) -> ()  [unwired: 1 in, 2 out]
      }
      event User Event {
        n417 = event-data() -> ("SelfPrint"=w1045:string)  [unwired: 1 in]
        n418 = Unbundle By Name(w1040) -> ("类别"=w1035:refnum<vi>, "PModel"=w1041:refnum<vi>, "大箱内产品"=w1042:refnum<vi>, "Adress"=w1034:refnum<vi>, "料号"=w1033:refnum<vi>)
        n419 = case shown="\"BarPrint\"" w1045 {
          tunnel: w1044 -> [w1048 w1078]
          tunnel: [w1048 w1067] -> w1043
          tunnel: w1042 -> [_ w1079]
          tunnel: w1041 -> [_ w1077]
          tunnel: w1040 -> [_ w1068]
          tunnel: [w1047 w1066] -> w1039
          tunnel: w1038 -> [w1047 _]
          tunnel: w1037 -> [w1046 w1065]
          tunnel: [w1046 w1064] -> w1036
          tunnel: w1035 -> [_ _]
          tunnel: w1034 -> [_ w1055]
          tunnel: w1033 -> [_ w1052]
          frame "假", Default {
          }
          frame "BarPrint" {
            n420 = property class="Ring (严格)"(reference=w1077) -> ("RingText.Text"=w1058:string)  [unwired: 1 in, 2 out]
            n421 = property class="Str"(reference=w1079, error in=w1078) -> (error out=w1063:errorcluster, "Text.Text"=w1062:string)  [unwired: 1 out]
            n422 = property class="Str"(reference=w1055) -> ("Value"=w1054:string)  [unwired: 1 in, 2 out]
            n423 = property class="Str"(reference=w1052) -> ("Value"=w1051:string)  [unwired: 1 in, 2 out]
            n424 = call "StrToArray.vi"("error in"=w1063, "StrIn"=w1062) -> ("error out"=w1060:errorcluster, "ArrayOut"=w1059:string[])  [unwired: 8 in]
            n425 = Concatenate Strings("地址：", w1054, "\n", "料号：", w1051) -> (w1050:string)
            n426 = call "BTxtFlash.vi"("error in"=w1060, "Model"=w1058, "ArrayIn"=w1059, "Path"="Config\\BigBox\\BSN2.txt") -> ("error out"=w1070:errorcluster)  [unwired: 7 in]
            n427 = call "BTxtFlash.vi"("error in"=w1060, "Model"=w1058, "ArrayIn"=w1059, "Path"="Config\\BigBox\\BModel.txt") -> ("error out"=w1072:errorcluster)  [unwired: 7 in]
            n428 = call "BTxtFlash.vi"("error in"=w1060, "Model"=w1058, "ArrayIn"=w1059, "Path"="Config\\BigBox\\BSN1.txt") -> ("error out"=w1071:errorcluster)  [unwired: 7 in]
            n429 = call "BTxtFlash.vi"("BAdress"=w1050, "error in"=w1060, "Model"=w1058, "ArrayIn"=w1059, "Path"="Config\\BigBox\\BAdress.txt") -> ("error out"=w1049:errorcluster)  [unwired: 6 in]
            n430 = call "BTxtFlash.vi"("error in"=w1060, "Model"=w1058, "ArrayIn"=w1059, "Path"="Config\\BigBox\\BDate.txt") -> ("error out"=w1074:errorcluster)  [unwired: 7 in]
            n431 = call "BTxtFlash.vi"("error in"=w1060, "Model"=w1058, "ArrayIn"=w1059, "Path"="Config\\BigBox\\BNumber.txt") -> ("error out"=w1073:errorcluster)  [unwired: 7 in]
            n432 = Merge Errors(w1074, w1073, w1072, w1071, w1070, w1049) -> (w1075:errorcluster)
            n433 = call "StickerPrint.vi"("error in"=w1075, "Path"="Config\\BigBox\\102152.btw") -> ("error out"=w1069:errorcluster)  [unwired: 9 in]
            n434 = flat-sequence {
              tunnel: w1069 -> [w1089]
              tunnel: w1068 -> [w1096]
              tunnel: [w1088] -> w1067
              tunnel: [w1087] -> w1066
              tunnel: w1065 -> [_]
              tunnel: [0] -> w1064
              frame #0 {
                w1087 = ""
                w1093 = 0
                n435 = Unbundle By Name(w1096) -> ("设定大箱总数"=w1095:refnum<vi>, "当前大箱内数量"=w1094:refnum<vi>, "大箱内产品"=w1092:refnum<vi>, "条码"=w1091:refnum<vi>)
                n436 = property class="DigNum (严格)"(reference=w1095, "DisabledEnum"=w1093) -> ()  [unwired: 1 in, 2 out]
                n437 = property class="DigNum (严格)"(reference=w1094, "Value"=w1093) -> ()  [unwired: 1 in, 2 out]
                n438 = property class="Str"(reference=w1092, error in=w1089, "Text.Text"=w1087) -> (error out=w1088:errorcluster)  [unwired: 1 out]
                n439 = property class="Str"(reference=w1091, "Text.Text"=w1087, "Key Focus"=TRUE, "DisabledEnum"=0) -> ()  [unwired: 1 in, 2 out]
              }
            }
          }
        }
      }
      event "类别": Value Change {
        n440 = event-data() -> ("CtlRef"=w1101:refnum<vi>)  [unwired: 1 in]
        n441 = Unbundle By Name(w1100) -> ("PModel"=w1099:refnum<vi>)
        n442 = disable-structure shown="启用" {
          disable-tunnel: w1101 -> [w1108 w1120]
          disable-tunnel: w1099 -> [w1107 w1117]
          disable-tunnel: w1098 -> [w1105 w1111]
          disable-tunnel: [w1104 w1109] -> w1097
          frame Disabled {
            n443 = call "GetExportModel.vi"("error in"=w1105, "型号"=w1107, "Debug"=FALSE, "产品类型"=w1108) -> ("error out"=w1104:errorcluster)  [unwired: 7 in]
          }
          frame Enabled {
            n444 = property class="Ring (严格)"(reference=w1120) -> ("RingText.Text"=w1119:string)  [unwired: 1 in, 2 out]
            n445 = Equal?(x=w1119, y="自产") -> (x = y?=w1115:bool)
            n446 = Select(t="Config\\data.ini" ("Path"), s=w1115, f="Config\\BSJ.ini" ("Path")) -> (s? t:f=w1112:string)
            n447 = call "Choice Dev.vi"("error in"=w1111, "Path"=w1112) -> ("error out"=w1110:errorcluster, "model"=w1116:string[])  [unwired: 6 in, 1 out]
            n448 = property class="Ring (严格)"(reference=w1117, error in=w1110, "Strings []"=w1116) -> (error out=w1109:errorcluster)  [unwired: 1 out]
          }
        }
      }
      event "PModel": Value Change {
        n449 = event-data() -> ("CtlRef"=w1127:refnum<vi>)  [unwired: 1 in]
        n450 = Unbundle By Name(w1131) -> ("类别"=w1130:refnum<vi>)
        n451 = property class="Ring (严格)"(reference=w1130) -> ("RingText.Text"=w1129:string)  [unwired: 1 in, 2 out]
        n452 = property class="Ring (严格)"(reference=w1127) -> ("Value"=w1123:u16)  [unwired: 1 in, 2 out]
        n453 = Equal?(x=w1129, y="自产") -> (x = y?=w1122:bool)
        n454 = Select(t=w1126, s=w1122, f=w1125) -> (s? t:f=w1124:string[][])
        n455 = Index Array(array=w1124, index (row)=w1123) -> (element=w1121:string[])  [unwired: 1 in]
        n456 = case shown="真" w1122 {
          tunnel: w1121 -> [w1135 w1136]
          frame False {
            n457 = global write "GlobalV.vi" "BSJMode"(w1135) -> ()
          }
          frame True {
            n458 = global write "GlobalV.vi" "SelfMode"(w1136) -> ()
          }
        }
      }
      event "清空": Value Change {
        n459 = event-data() -> ("CtlRef"=w1147:refnum<vi>, "NewVal"=w1146:bool)  [unwired: 1 in]
        n460 = Unbundle By Name(w1139) -> ("当前大箱内数量"=w1138:refnum<vi>, "大箱内产品"=w1137:refnum<vi>)
        n461 = case shown="假" w1146 {
          tunnel: w1147 -> [w1151 w1158]
          tunnel: w1145 -> [w1149 _]
          tunnel: w1144 -> [w1150 _]
          tunnel: [w1151 w1158] -> w1143
          tunnel: [w1150 0] -> w1141
          tunnel: [w1149 ""] -> w1140
          tunnel: w1138 -> [_ w1155]
          tunnel: w1137 -> [_ w1154]
          frame False {
          }
          frame True {
            n462 = property class="Str"(reference=w1154, "Text.Text"="") -> ()  [unwired: 1 in, 2 out]
            n463 = property class="DigNum (严格)"(reference=w1155, "Value"=0) -> ()  [unwired: 1 in, 2 out]
          }
        }
        n464 = property class="Bool (严格)"(reference=w1143, "Value"=FALSE) -> ()  [unwired: 1 in, 2 out]
      }
    }
  }
  n465 = while {
    tunnel: w53 -> [w1174]
    tunnel: w52 -> [w1173]
    shift-right: [w1171] -> _
    shift-left: w51 -> [w1172]
    tunnel: w50 -> [w1169]
    tunnel: w1 -> [w1168]
    tunnel: w49 -> [w1167]
    tunnel: w48 -> [w1166]
    tunnel: w3 -> [w1165]
    tunnel: w47 -> [w1164]
    tunnel: w46 -> [w1163]
    tunnel: w45 -> [w1162]
    tunnel: w3 -> [w1161]
    tunnel: [w1160] -> w20
    tunnel: [w1159] -> w24
    stop <- w1170 stop-if-true
    # "BSJ包装循环"
    n466 = event shown="[1] \"数据导入\": 值改变" {
      selector: w1174 -> [_ _ _ _ _ _ _ _]
      dyn-events: [_ _ _ _ _ _ _ _] -> w1159
      timeout: 20 -> [_ _ _ _ _ _ _ _]
      tunnel: w1173 -> [_ w1188 _ _ _ _ _ _]
      tunnel: w1172 -> [w1177 w1187 w1222 w1232 w1237 w1386 w1424 w1498]
      tunnel: [w1177 w1184 w1222 w1232 w1237 w1386 w1424 w1498] -> w1171
      tunnel: [w1178 _ _ _ _ _ _ _] -> w1170
      tunnel: w1169 -> [_ w1183 _ _ w1240 _ w1422 w1493]
      tunnel: w1168 -> [_ _ w1225 _ _ _ _ _]
      tunnel: w1167 -> [_ _ w1224 _ _ _ _ _]
      tunnel: w1166 -> [w1176 w1180 w1221 w1231 w1243 w1390 w1419 w1494]
      tunnel: w1165 -> [_ _ _ w1235 w1242 w1385 w1421 _]
      tunnel: w1164 -> [_ w1182 _ _ _ _ _ _]
      tunnel: w1163 -> [_ _ _ _ w1247 w1387 _ _]
      tunnel: w1162 -> [_ _ _ _ _ w1391 _ w1495]
      tunnel: w1161 -> [_ _ _ _ _ _ w1416 _]
      tunnel: [w1176 w1179 w1220 w1230 w1236 w1390 w1417 w1489] -> w1160
      event Timeout {
        n467 = event-data() -> ()  [unwired: 1 in, 3 out]
        n468 = global read "GlobalV.vi" "Stop"() -> (w1178:bool)
      }
      event "数据导入": Value Change {
        n469 = event-data() -> ("CtlRef"=w1186:refnum<vi>)  [unwired: 1 in]
        n470 = property class="Ring (严格)"(reference=w1183, error in=w1180) -> (error out=w1181:errorcluster, "RingText.Text"=w1192:string)  [unwired: 1 out]
        n471 = property class="Str"(reference=w1188, "Value"="") -> (reference out=w1190:refnum<vi>)  [unwired: 1 in, 1 out]
        n472 = call "RecordPath.vi"("error in"=w1181, "Path"="Config\\出货清单.xls") -> ("error out"=w1196:errorcluster, "PathOut"=w1197:path)  [unwired: 8 in]
        n473 = Format Date/Time String(time format string (%c)="%Y-%m-%d %H:%M:%S" ("时间格式字符串(%c)")) -> (date/time string=w1191:string)  [unwired: 2 in]
        n474 = call "ReadExcel.vi"("error in"=w1196, "template"=w1197) -> ("error out"=w1194:errorcluster, "data"=w1195:string[][])  [unwired: 8 in]
        n475 = for {
          tunnel: w1195 -> [w1210] mode=indexing
          tunnel: w1194 -> [w1205]
          tunnel: w1192 -> [w1209]
          tunnel: w1191 -> [w1208]
          shift-right: [w1212] -> w1184
          shift-left: w1187 -> [w1216]
          tunnel: w1190 -> [w1217]
          tunnel: [w1211] -> w1185
          tunnel: w1182 -> [w1207]
          i -> [w1215]
          n476 = case shown="1, 默认" w1215 {
            tunnel: ["" "\n"] -> w1214
            frame 0 {
            }
            frame 1, Default {
            }
          }
          n477 = call "RecordIntoDB.vi"("Debug"=FALSE, "Model"=w1209, "error in"=w1205, "Time"=w1208, "产品类别"=w1207, "ArrayIn"=w1210) -> ("error out"=w1203:errorcluster, "Result"=w1204:string)  [unwired: 4 in]
          n478 = Concatenate Strings(w1216, w1214, w1204) -> (w1212:string)
          n479 = String Length(string=w1212) -> (length=w1213:i32)
          n480 = property class="Str"(reference=w1217, error in=w1203, "Text.Text"=w1212, "Text.Scroll Position"=w1213) -> (error out=w1211:errorcluster)  [unwired: 1 out]
        }
        n481 = flat-sequence {
          tunnel: w1186 -> [w1202]
          tunnel: w1185 -> [w1201]
          tunnel: [w1199] -> w1179
          frame #0 {
            n482 = property class="Bool (严格)"(reference=w1202, error in=w1201, "Value"=FALSE) -> (error out=w1199:errorcluster)  [unwired: 1 out]
          }
        }
      }
      event "BSJ型号": Value Change {
        n483 = event-data() -> ("CtlRef"=w1226:refnum<vi>)  [unwired: 1 in]
        n484 = property class="Ring (严格)"(reference=w1226, error in=w1221) -> (error out=w1227:errorcluster, "Value"=w1229:u16)  [unwired: 1 out]
        n485 = Index Array(array=w1225, index (row)=w1229) -> (element=w1223:string[])  [unwired: 1 in]
        n486 = global write "GlobalV.vi" "BSJMode"(w1223) -> ()
        n487 = Index Array(array=w1223) -> (element=w1228:string)  [unwired: 1 in]
        n488 = property class="Str"(reference=w1224, error in=w1227, "Value"=w1228) -> (error out=w1220:errorcluster)  [unwired: 1 out]
      }
      event "能未满封箱？": Value Change {
        n489 = event-data() -> ("NewVal"=w1233:bool)  [unwired: 1 in]
        n490 = Unbundle By Name(w1235) -> ("人工封箱"=w1234:refnum<vi>)
        n491 = property class="Bool (严格)"(reference=w1234, error in=w1231, "Value"=w1233) -> (error out=w1230:errorcluster)  [unwired: 1 out]
      }
      event "SN码": Value Change {
        n492 = event-data() -> ("NewVal"=w1259:string)  [unwired: 1 in]
        n493 = global read "GlobalV.vi" "BSJMode"() -> (w1258:string[])
        n494 = property class="Ring (严格)"(reference=w1240) -> ("RingText.Text"=w1239:string)  [unwired: 1 in, 2 out]
        n495 = Unbundle By Name(w1242) -> ("SN码"=w1246:refnum<vi>)
        n496 = call <vilib>:"Trim Whitespace.vi"("string"=w1259) -> ("trimmed string"=w1260:string)  [unwired: 1 in]
        n497 = Index Array(array=w1258, index #2=1 ("索引"), index #3=2 ("索引")) -> (element #1=w1251:string, element #2=w1255:string, element #3=w1248:string)  [unwired: 1 in]
        n498 = String Length(string=w1248) -> (length=w1249:i32)
        n499 = Unbundle By Name(w1242) -> ("BSJ产品记录"=w1241:refnum<vi>)
        n500 = Decimal String To Number(string=w1255) -> (number=w1254:i32)  [unwired: 2 in, 1 out]
        n501 = String Subset(string=w1260, length (rest)=w1249) -> (substring=w1261:string)  [unwired: 1 in]
        n502 = String Length(string=w1260) -> (length=w1238:i32)
        n503 = property class="Str"(reference=w1246, "DisabledEnum"=2) -> (reference out=w1245:refnum<vi>)  [unwired: 1 in, 1 out]
        n504 = Equal?(x=w1238, y=w1254) -> (x = y?=w1253:bool)
        n505 = Equal?(x=w1261, y=w1248) -> (x = y?=w1252:bool)
        n506 = And(x=w1253, y=w1252) -> (x .and. y?=w1244:bool)
        n507 = case shown="真" w1244 {
          tunnel: w1245 -> [w1271 w1293]
          tunnel: w1238 -> [w1270 _]
          tunnel: w1255 -> [w1269 _]
          tunnel: w1248 -> [w1268 _]
          tunnel: w1260 -> [_ w1298]
          tunnel: w1241 -> [_ w1291]
          tunnel: w1251 -> [_ w1290]
          tunnel: w1247 -> [_ w1289]
          tunnel: w1243 -> [w1267 w1288]
          tunnel: [w1263 w1286] -> w1236
          tunnel: w1239 -> [_ w1285]
          frame False {
            n508 = flat-sequence {
              tunnel: w1270 -> [w1283]
              tunnel: w1269 -> [w1279]
              tunnel: [w1277] -> w1272
              tunnel: w1271 -> [w1277]
              tunnel: w1268 -> [w1275]
              frame #0 {
                n509 = Number To Decimal String(number=w1283) -> (decimal integer string=w1281:string)  [unwired: 1 in]
                n510 = Concatenate Strings("条码长度或前置规则不匹配，请检查后重试！\n" ("消息"), "实际条码长度 ", w1281, "，要求条码长度 ", w1279, "\n前置规则要求：" ("字符串"), w1275) -> (w1278:string)
                n511 = One Button Dialog(message=w1278) -> ()  [unwired: 1 in, 1 out]
              }
            }
            n512 = property class="Str"(reference=w1272, error in=w1267, "Key Focus"=TRUE ("键选中"), "DisabledEnum"=0, "Value"="") -> (reference out=w1264:refnum<vi>, error out=w1265:errorcluster)
            n513 = property class="Str"(reference=w1264, error in=w1265, "Key Focus"=TRUE ("键选中")) -> (error out=w1263:errorcluster)  [unwired: 1 out]
          }
          frame True {
            n514 = Concatenate Strings("'" ("字符串"), w1285, "','" ("字符串"), w1298, "',@A" ("字符串")) -> (w1297:string)
            n515 = call "DBGetData.vi"("error in"=w1288, "String"=w1297, "Procedure"="prc_BSJPackGetdata") -> ("error out"=w1287:errorcluster, "Data Out"=w1295:string[][])  [unwired: 7 in]
            n516 = Index Array(array=w1295) -> (element=w1292:string[])  [unwired: 2 in]
            n517 = Array Size(array=w1292) -> (size(s)=w1294:i32)
            n518 = case shown="1" w1294 {
              tunnel: w1293 -> [w1304 w1321 w1344]
              tunnel: w1292 -> [_ w1322 w1345]
              tunnel: w1291 -> [_ _ w1346]
              tunnel: w1290 -> [_ _ w1343]
              tunnel: w1289 -> [_ _ w1342]
              tunnel: w1287 -> [w1303 w1320 w1341]
              tunnel: [w1302 w1318 w1337] -> w1286
              frame -1, 0, Default {
                n519 = flat-sequence {
                  tunnel: w1304 -> [w1306]
                  tunnel: [w1306] -> w1305
                  tunnel: w1305 -> [w1315]
                  tunnel: w1303 -> [w1314]
                  tunnel: [w1312] -> w1302
                  frame #0 {
                    n520 = One Button Dialog(message="您输入的SN未通过测试！\n或\n外部条码与内部条码不一致，请检查！" ("消息")) -> ()  [unwired: 1 in, 1 out]
                  }
                  frame #1 {
                    n521 = property class="Str"(reference=w1315, error in=w1314, "Value"="", "DisabledEnum"=T3."Enabled" ("禁用")) -> (reference out=w1311:refnum<vi>, error out=w1313:errorcluster)
                    n522 = property class="Str"(reference=w1311, error in=w1313, "Key Focus"=TRUE ("键选中")) -> (error out=w1312:errorcluster)  [unwired: 1 out]
                  }
                }
              }
              frame 1 {
                n523 = flat-sequence {
                  tunnel: w1322 -> [w1326]
                  tunnel: w1321 -> [w1324]
                  tunnel: [w1324] -> w1323
                  tunnel: w1323 -> [w1333]
                  tunnel: w1320 -> [w1329]
                  tunnel: [w1328] -> w1319
                  tunnel: [w1327] -> w1317
                  frame #0 {
                    n524 = Index Array(array=w1326) -> (element=w1325:string)  [unwired: 1 in]
                    n525 = One Button Dialog(message=w1325) -> ()  [unwired: 1 in, 1 out]
                  }
                  frame #1 {
                    n526 = property class="Str"(reference=w1333, error in=w1329, "Key Focus"=TRUE ("键选中"), "Value"="", "DisabledEnum"=T3."Enabled" ("禁用")) -> (reference out=w1327:refnum<vi>, error out=w1328:errorcluster)
                  }
                }
                n527 = property class="Str"(reference=w1317, error in=w1319, "Key Focus"=TRUE ("键选中")) -> (error out=w1318:errorcluster)  [unwired: 1 out]
              }
              frame 2..8 {
                n528 = flat-sequence {
                  tunnel: [w1377] -> w1354
                  tunnel: [w1376] -> w1353
                  tunnel: [w1375] -> w1350
                  tunnel: [w1374] -> w1352
                  tunnel: [w1368] -> w1349
                  tunnel: [w1371] -> w1348
                  tunnel: [w1366] -> w1347
                  tunnel: w1346 -> [w1370]
                  tunnel: w1345 -> [w1369]
                  tunnel: w1344 -> [w1368]
                  tunnel: w1343 -> [w1367]
                  tunnel: w1342 -> [w1366]
                  tunnel: w1341 -> [w1365]
                  tunnel: [w1364] -> w1340
                  frame #0 {
                    n529 = property class="MCListbox (严格)"(reference=w1370, error in=w1365) -> (reference out=w1377:refnum<vi>, error out=w1364:errorcluster, "ItemNames"=w1379:string[][])
                    n530 = Decimal String To Number(string=w1367) -> (number=w1372:i32)  [unwired: 2 in, 1 out]
                    n531 = Array Size(array=w1379) -> (size(s)=w1380:i32[])
                    n532 = Insert Into Array(array=w1379, new element=w1369) -> (w1374:string[][])  [unwired: 2 in]
                    n533 = Index Array(array=w1380) -> (element=w1381:i32)  [unwired: 1 in]
                    n534 = Increment(x=w1381) -> (x+1=w1373:i32)
                    n535 = for {
                      N: w1373 -> [_]
                      tunnel: [w1382] -> w1378 mode=indexing
                      tunnel: [w1383] -> w1375
                      i -> [w1383]
                      n536 = Increment(x=w1383) -> (x+1=w1382:i32)
                    }
                    n537 = Greater Or Equal?(x=w1373, y=w1372) -> (x >= y?=w1371:bool)
                    n538 = Number To Decimal String(number=w1378) -> (decimal integer string=w1376:string[])  [unwired: 1 in]
                  }
                }
                n539 = call "TopLeft position.vi"("index"=w1350) -> ("TopLeft"=w1351:T4)
                n540 = property class="MCListbox (严格)"(reference=w1354, error in=w1340, "RowHdrs[]"=w1353, "Value"=w1350, "ItemNames"=w1352, "TopLeft"=w1351) -> (error out=w1339:errorcluster)  [unwired: 1 out]
                n541 = property class="Str"(reference=w1349, error in=w1339, "Value"="", "DisabledEnum"=0) -> (reference out=w1334:refnum<vi>, error out=w1338:errorcluster)
                n542 = case shown="假" w1348 {
                  tunnel: w1347 -> [_ w1363]
                  tunnel: w1338 -> [w1357 w1361]
                  tunnel: [w1357 w1360] -> w1337
                  tunnel: w1334 -> [w1356 w1359]
                  frame False {
                    n543 = property class="Str"(reference=w1356, "Key Focus"=TRUE) -> ()  [unwired: 1 in, 2 out]
                  }
                  frame True {
                    n544 = property class="Str"(reference=w1359, "Key Focus"=TRUE ("键选中")) -> ()  [unwired: 1 in, 2 out]
                    n545 = Generate User Event(user event=w1363, event data cluster="WriteDataToDB" ("事件数据"), error in=w1361) -> (error out=w1360:errorcluster)  [unwired: 1 in, 1 out]
                  }
                }
              }
            }
          }
        }
      }
      event "人工封箱": Value Change {
        n546 = event-data() -> ("CtlRef"=w1389:refnum<vi>, "NewVal"=w1388:bool)  [unwired: 1 in]
        n547 = property class="MCListbox (严格)"(reference=w1391, error in=w1390) -> (error out=w1393:errorcluster, "ItemNames"=w1396:string[][])  [unwired: 1 out]
        n548 = Unbundle By Name(w1385) -> ("SN码"=w1384:refnum<vi>)
        n549 = case shown="假" w1388 {
          tunnel: w1389 -> [w1398 w1402]
          tunnel: w1396 -> [_ w1409]
          tunnel: w1387 -> [_ w1404]
          tunnel: w1384 -> [_ w1403]
          tunnel: [w1398 w1402] -> w1394
          tunnel: w1393 -> [w1397 w1401]
          tunnel: [w1397 w1400] -> w1392
          frame False {
          }
          frame True {
            n550 = Array Size(array=w1409) -> (size(s)=w1408:i32[])
            n551 = Index Array(array=w1408) -> (element=w1407:i32)  [unwired: 1 in]
            n552 = property class="Str"(reference=w1403, "Value"="") -> ()  [unwired: 1 in, 2 out]
            n553 = Greater Or Equal?(x=w1407, y=1) -> (x >= y?=w1405:bool)
            n554 = case shown="真" w1405 {
              tunnel: w1404 -> [_ w1412]
              tunnel: w1401 -> [w1410 w1414]
              tunnel: [w1410 w1413] -> w1400
              frame False {
                n555 = One Button Dialog(message="包装箱数据为空！" ("消息")) -> ()  [unwired: 1 in, 1 out]
              }
              frame True {
                n556 = Generate User Event(user event=w1412, event data cluster="WriteDataToDB" ("事件数据"), error in=w1414) -> (error out=w1413:errorcluster)  [unwired: 1 in, 1 out]
              }
            }
          }
        }
        n557 = property class="Bool (严格)"(reference=w1394, error in=w1392, "Value"=FALSE ("值")) -> ()  [unwired: 2 out]
      }
      event User Event {
        n558 = event-data() -> ("PackEve"=w1423:string)  [unwired: 1 in]
        n559 = Unbundle By Name(w1416) -> ("客户地址"=w1418:refnum<vi>)
        n560 = Unbundle By Name(w1421) -> ("BSJ产品记录"=w1420:refnum<vi>)
        n561 = case shown="\"WriteDataToDB\"" w1423 {
          tunnel: w1420 -> [_ w1456]
          tunnel: w1422 -> [_ w1441]
          tunnel: w1418 -> [_ w1440]
          tunnel: w1419 -> [w1425 w1437]
          tunnel: [w1425 w1436] -> w1417
          frame "假", Default {
          }
          frame "WriteDataToDB" {
            w1452 = ","
            w1442 = "'"
            n562 = property class="MCListbox (严格)"(reference=w1456, error in=w1437) -> (reference out=w1444:refnum<vi>, error out=w1431:errorcluster, "ItemNames"=w1428:string[][])
            n563 = property class="Ring (严格)"(reference=w1441) -> ("RingText.Text"=w1427:string)  [unwired: 1 in, 2 out]
            n564 = Format Date/Time String(time format string (%c)="%Y%m%d" ("时间格式字符串(%c)")) -> (date/time string=w1434:string)  [unwired: 2 in]
            n565 = property class="Str"(reference=w1440) -> ("Value"=w1439:string)  [unwired: 1 in, 2 out]
            n566 = String Subset(string=w1434, offset (0)=2 ("偏移量(0)")) -> (substring=w1432:string)  [unwired: 1 in]
            n567 = for {
              tunnel: w1428 -> [w1488] mode=indexing
              shift-right: [w1485] -> w1453
              shift-left: "" -> [w1487]
              n568 = Index Array(array=w1488, index=3 ("索引")) -> (element=w1486:string)
              n569 = Concatenate Strings(w1487, w1486, ",") -> (w1485:string)
            }
            n570 = call "GetBoxNo.vi"("error in"=w1431, "种类"=enum16{"自产", "外购"}."外购", "TimeStr"=w1432, "Model"=w1427) -> ("error out"=w1430:errorcluster, "BoxNo"=w1429:string)  [unwired: 6 in]
            n571 = String Length(string=w1453) -> (length=w1454:i32)
            n572 = Decrement(x=w1454) -> (x-1=w1455:i32)
            n573 = String Subset(string=w1453, length (rest)=w1455) -> (substring=w1438:string)  [unwired: 1 in]
            n574 = Concatenate Strings(w1442, w1427, w1442, w1452, w1442, w1429, w1442, w1452, w1442, w1439, w1442, w1452, w1442, w1438, w1442, w1452, "@A" ("字符串")) -> (w1450:string)
            n575 = call "prc_writeBOXdata.vi"("string"=w1450, "Process"="prc_BSJPackaged") -> ("Array"=w1448:string[][])  [unwired: 8 in, 1 out]
            n576 = Index Array(array=w1448) -> (element=w1447:string[])  [unwired: 2 in]
            n577 = Index Array(array=w1447) -> (element=w1443:string)  [unwired: 1 in]
            n578 = Equal?(x=w1443, y="OK") -> (x = y?=w1445:bool)
            n579 = case shown="假" w1445 {
              tunnel: w1444 -> [_ w1482]
              tunnel: w1443 -> [w1459 _]
              tunnel: w1430 -> [w1458 w1470]
              tunnel: [w1458 w1461] -> w1436
              tunnel: w1428 -> [_ w1471]
              tunnel: w1427 -> [_ w1469]
              frame False {
                n580 = One Button Dialog(message=w1459) -> ()  [unwired: 1 in, 1 out]
              }
              frame True {
                w1460 = 3 ("Index")
                n581 = invoke class="MCListbox (严格)" method="Reinit To Default"(reference=w1482, error in=w1470) -> (reference out=w1481:refnum<vi>, error out=w1477:errorcluster)  [unwired: 1 in, 1 out]
                n582 = call "TxtFlash.vi"("Index"=w1460, "error in"=w1470, "Model"=w1469, "ItemNames"=w1471, "Path"="Config\\MidBox\\Date.txt") -> ("error out"=w1468:errorcluster)  [unwired: 6 in]
                n583 = call "TxtFlash.vi"("Index"=w1460, "error in"=w1470, "Model"=w1469, "ItemNames"=w1471, "Path"="Config\\MidBox\\Number.txt") -> ("error out"=w1467:errorcluster)  [unwired: 6 in]
                n584 = call "TxtFlash.vi"("Index"=w1460, "error in"=w1470, "Model"=w1469, "ItemNames"=w1471, "Path"="Config\\MidBox\\SN.txt") -> ("error out"=w1466:errorcluster)  [unwired: 6 in]
                n585 = call "TxtFlash.vi"("Index"=w1460, "error in"=w1470, "Model"=w1469, "ItemNames"=w1471, "Path"="Config\\MidBox\\Model.txt") -> ("error out"=w1465:errorcluster)  [unwired: 6 in]
                n586 = property class="MCListbox (严格)"(reference=w1481, error in=w1477, "SelColor"=u32 16775631, "RowHdrs[]"=string[] [] ("行首字符串[]"), "ItemNames"=string[][] [] ("项名")) -> (error out=w1462:errorcluster)  [unwired: 1 out]
                n587 = Merge Errors(w1468, w1467, w1466, w1465) -> (w1464:errorcluster)
                n588 = call "StickerPrint.vi"("error in"=w1464, "Path"="Config\\MidBox\\58102.btw") -> ("error out"=w1463:errorcluster)  [unwired: 9 in]
                n589 = Merge Errors(w1463, w1462) -> (w1461:errorcluster)
              }
            }
          }
        }
      }
      event "删除单个数据": Value Change {
        n590 = event-data() -> ("CtlRef"=w1497:refnum<vi>, "NewVal"=w1496:bool)  [unwired: 1 in]
        n591 = case shown="真" w1496 {
          tunnel: w1497 -> [w1500 w1535]
          tunnel: [w1500 w1535] -> w1492
          tunnel: w1495 -> [_ w1534]
          tunnel: w1493 -> [_ w1518]
          tunnel: w1494 -> [w1499 w1504]
          tunnel: [w1499 w1501] -> w1490
          frame False {
          }
          frame True {
            n592 = property class="MCListbox (严格)"(reference=w1534, error in=w1504) -> (reference out=w1523:refnum<vi>, error out=w1503:errorcluster, "ItemNames"=w1532:string[][], "Value"=w1530:i32)
            n593 = property class="Ring (严格)"(reference=w1518) -> ("RingText.Text"=w1516:string)  [unwired: 1 in, 2 out]
            n594 = Greater Or Equal To 0?(x=w1530) -> (x >= 0?=w1529:bool)
            n595 = Delete From Array(array=w1532, length=1 ("长度"), index (row)=w1530) -> (deleted portion=w1517:string[][], array with subset deleted=w1520:string[][])  [unwired: 1 in]
            n596 = Index Array(array=w1517, index (row)=0 ("索引 (行)"), index (col)=3 ("禁用的索引 (列)")) -> (element=w1515:string)
            n597 = Array Size(array=w1532) -> (size(s)=w1531:i32[])
            n598 = Build Array(w1516, w1515) -> (w1512:string[])
            n599 = Index Array(array=w1531) -> (element=w1527:i32)  [unwired: 1 in]
            n600 = for {
              tunnel: w1512 -> [w1539] mode=indexing
              shift-right: [w1536] -> w1509
              shift-left: "" -> [w1540]
              w1538 = "'" ("字符串")
              n601 = Concatenate Strings(w1540, w1538, w1539, w1538, "," ("字符串")) -> (w1536:string)
            }
            n602 = Decrement(x=w1527) -> (x-1=w1528:i32)
            n603 = Select(t=w1528, s=w1529, f=w1527) -> (s? t:f=w1526:i32)
            n604 = for {
              N: w1526 -> [_]
              tunnel: [w1542] -> w1524 mode=indexing
              tunnel: [w1541] -> w1525
              i -> [w1541]
              n605 = Increment(x=w1541) -> (x+1=w1542:i32)
            }
            n606 = Concatenate Strings(w1509, "@A" ("字符串")) -> (w1511:string)
            n607 = call "TopLeft position.vi"("index"=w1525) -> ("TopLeft"=w1522:T4)
            n608 = call "prc_SetPackaged.vi"("error in"=w1503, "string"=w1511, "SQL query"="prc_BSJResetPackFlag") -> ("error out"=w1502:errorcluster, "Array"=w1508:string[][])  [unwired: 7 in]
            n609 = Number To Decimal String(number=w1524) -> (decimal integer string=w1521:string[])  [unwired: 1 in]
            n610 = Index Array(array=w1508) -> (element=w1507:string[])  [unwired: 2 in]
            n611 = Index Array(array=w1507) -> (element=w1506:string)  [unwired: 1 in]
            n612 = property class="MCListbox (严格)"(reference=w1523, error in=w1502, "RowHdrs[]"=w1521, "ItemNames"=w1520, "TopLeft"=w1522) -> (error out=w1501:errorcluster)  [unwired: 1 out]
            n613 = One Button Dialog(message=w1506) -> ()  [unwired: 1 in, 1 out]
          }
        }
        n614 = property class="Bool (严格)"(reference=w1492, error in=w1490, "Value"=FALSE) -> (error out=w1489:errorcluster)  [unwired: 1 out]
      }
    }
  }
  n615 = while {
    tunnel: w44 -> [w1557]
    tunnel: w43 -> [w1556]
    tunnel: w42 -> [w1555]
    tunnel: w41 -> [w1554]
    tunnel: w40 -> [w1553]
    tunnel: w39 -> [w1552]
    tunnel: w3 -> [w1551]
    tunnel: w38 -> [w1550]
    tunnel: w37 -> [w1549]
    tunnel: w36 -> [w1548]
    shift-right: [w1545] -> _
    shift-left: w35 -> [w1547]
    tunnel: w34 -> [w1546]
    tunnel: [w1544] -> w23
    tunnel: [w1543] -> w19
    stop <- w1558 stop-if-true
    # "出货及数据记录导出循环"
    n616 = event shown="[6] <ExportEve>: 用户事件" {
      selector: w1555 -> [_ _ _ _ _ _ _ _ _ _]
      dyn-events: [_ _ _ _ _ _ _ _ _ _] -> w1544
      timeout: 20 -> [_ _ _ _ _ _ _ _ _ _]
      tunnel: [w1562 _ _ _ _ _ _ _ _ _] -> w1558
      tunnel: w1557 -> [_ w1567 _ _ _ _ _ _ _ _]
      tunnel: w1556 -> [_ _ w1572 _ _ _ _ _ _ w2125]
      tunnel: w1554 -> [w1560 w1564 w1569 w1575 w1621 w1678 w2003 w2081 w2111 w2114]
      tunnel: w1553 -> [_ _ _ _ _ _ _ _ _ w2126]
      tunnel: w1552 -> [_ _ _ _ _ _ w2001 _ _ _]
      tunnel: w1551 -> [_ _ _ _ _ w1677 w2005 _ _ w2120]
      tunnel: w1550 -> [_ _ _ _ _ w1674 _ w2087 _ _]
      tunnel: w1549 -> [_ _ _ _ _ _ w2007 w2090 _ _]
      tunnel: w1548 -> [_ _ _ _ _ _ w2006 _ _ _]
      tunnel: w1547 -> [w1561 w1565 w1570 w1576 w1622 w1670 w2004 w2082 _ w2127]
      tunnel: w1546 -> [_ _ _ _ _ _ _ _ w2112 _]
      tunnel: [w1560 w1563 w1568 w1574 w1620 w1669 w2002 w2080 w2110 w2113] -> w1543
      tunnel: [w1561 w1565 w1570 w1576 w1622 w1670 w2004 w2082 w2109 w2127] -> w1545
      event Timeout {
        n617 = event-data() -> ()  [unwired: 1 in, 1 out]
        n618 = global read "GlobalV.vi" "Stop"() -> (w1562:bool)
      }
      event "出货方式": Value Change {
        n619 = event-data() -> ("NewVal"=w1566:bool)  [unwired: 1 in]
        n620 = property class="Bool (严格)"(reference=w1567, error in=w1564, "Visible"=w1566) -> (error out=w1563:errorcluster)  [unwired: 1 out]
      }
      event "产品种类": Value Change {
        n621 = event-data() -> ("CtlRef"=w1573:refnum<vi>)  [unwired: 1 in]
        n622 = call "GetExportModel.vi"("error in"=w1569, "型号"=w1572, "Debug"=FALSE, "产品类型"=w1573) -> ("error out"=w1568:errorcluster)  [unwired: 7 in]
      }
      event "设定出货数量": Value Change {
        n623 = event-data() -> ("NewVal"=w1577:string, "CtlRef"=w1578:refnum<vi>)  [unwired: 1 in]
        n624 = Empty String/Path?(string/path=w1577) -> (empty?=w1579:bool)
        n625 = case shown="假" w1579 {
          tunnel: w1577 -> [w1588 _]
          tunnel: w1578 -> [w1586 w1618]
          tunnel: w1577 -> [w1584 _]
          tunnel: w1575 -> [w1581 w1616]
          tunnel: [w1580 w1615] -> w1574
          frame False {
            n626 = flat-sequence {
              tunnel: w1588 -> [w1594]
              tunnel: [w1592] -> w1587
              tunnel: w1586 -> [w1591]
              tunnel: [w1591] -> w1585
              tunnel: w1584 -> [w1590]
              tunnel: [w1590] -> w1583
              tunnel: [w1589] -> w1582
              tunnel: w1581 -> [w1589]
              tunnel: w1587 -> [w1600]
              tunnel: w1585 -> [w1599]
              tunnel: w1583 -> [w1598]
              tunnel: w1582 -> [w1597]
              tunnel: [w1596] -> w1580
              frame #0 {
                n627 = Concatenate Strings("本次出货数量为：" ("消息"), w1594) -> (w1593:string)
                n628 = Two Button Dialog(message=w1593) -> (T button?=w1592:bool)  [unwired: 2 in]
              }
              frame #1 {
                n629 = case shown="假" w1600 {
                  tunnel: w1599 -> [w1608 w1614]
                  tunnel: w1598 -> [_ w1612]
                  tunnel: w1597 -> [w1605 w1611]
                  tunnel: [w1602 w1610] -> w1596
                  frame False {
                    n630 = property class="Str"(reference=w1608, error in=w1605, "DisabledEnum"=0, "Key Focus"=TRUE, "Value"="") -> (reference out=w1603:refnum<vi>, error out=w1604:errorcluster)
                    n631 = property class="Str"(reference=w1603, error in=w1604, "Key Focus"=TRUE) -> (error out=w1602:errorcluster)  [unwired: 1 out]
                  }
                  frame True {
                    n632 = property class="Str"(reference=w1614, error in=w1611, "DisabledEnum"=2, "Value"=w1612) -> (error out=w1610:errorcluster)  [unwired: 1 out]
                  }
                }
              }
            }
          }
          frame True {
            n633 = property class="Str"(reference=w1618, error in=w1616, "DisabledEnum"=0) -> (error out=w1615:errorcluster)  [unwired: 1 out]
            n634 = One Button Dialog(message="出货数量为空，请设置正确的出货数量！" ("消息")) -> ()  [unwired: 1 in, 1 out]
          }
        }
      }
      event "出货地址": Value Change {
        n635 = event-data() -> ("NewVal"=w1623:string, "CtlRef"=w1624:refnum<vi>)  [unwired: 1 in]
        n636 = Empty String/Path?(string/path=w1623) -> (empty?=w1625:bool)
        n637 = case shown="假" w1625 {
          tunnel: w1623 -> [w1634 _]
          tunnel: w1624 -> [w1632 w1660]
          tunnel: w1623 -> [w1630 _]
          tunnel: w1621 -> [w1627 w1659]
          tunnel: [w1626 w1658] -> w1620
          frame False {
            n638 = flat-sequence {
              tunnel: w1634 -> [w1640]
              tunnel: [w1638] -> w1633
              tunnel: w1632 -> [w1637]
              tunnel: [w1637] -> w1631
              tunnel: w1630 -> [w1636]
              tunnel: [w1636] -> w1629
              tunnel: [w1635] -> w1628
              tunnel: w1627 -> [w1635]
              tunnel: w1633 -> [w1646]
              tunnel: w1631 -> [w1645]
              tunnel: w1629 -> [w1644]
              tunnel: w1628 -> [w1643]
              tunnel: [w1642] -> w1626
              frame #0 {
                n639 = Concatenate Strings("本次出货地址为：" ("消息"), w1640) -> (w1639:string)
                n640 = Two Button Dialog(message=w1639) -> (T button?=w1638:bool)  [unwired: 2 in]
              }
              frame #1 {
                n641 = case shown="真" w1646 {
                  tunnel: w1645 -> [w1651 w1657]
                  tunnel: w1644 -> [_ w1655]
                  tunnel: w1643 -> [w1648 w1654]
                  tunnel: [w1647 w1653] -> w1642
                  frame False {
                    n642 = property class="Str"(reference=w1651, error in=w1648, "DisabledEnum"=0, "Key Focus"=TRUE, "Value"="") -> (error out=w1647:errorcluster)  [unwired: 1 out]
                  }
                  frame True {
                    n643 = property class="Str"(reference=w1657, error in=w1654, "DisabledEnum"=2, "Value"=w1655) -> (error out=w1653:errorcluster)  [unwired: 1 out]
                  }
                }
              }
            }
          }
          frame True {
            n644 = property class="Str"(reference=w1660, error in=w1659, "DisabledEnum"=0) -> (error out=w1658:errorcluster)  [unwired: 1 out]
            n645 = One Button Dialog(message="出货地址为空，请设置正确的出货地址！" ("消息")) -> ()  [unwired: 1 in, 1 out]
          }
        }
      }
      event "包装箱条码": Value Change {
        n646 = event-data() -> ("CtlRef"=w1673:refnum<vi>, "NewVal"=w1665:string)  [unwired: 1 in, 1 out]
        n647 = Unbundle By Name(w1677) -> ("产品种类"=w1667:refnum<vi>, "包装箱条码"=w1668:refnum<vi>, "箱内产品信息"=w1676:refnum<vi>, "设定出货数量"=w1675:refnum<vi>, "出货地址"=w1672:refnum<vi>, "设定出货数量"=w1671:refnum<vi>)
        n648 = Not Equal?(x=w1665, y="") -> (x != y?=w1663:bool)
        n649 = case shown="真" w1663 {
          tunnel: w1678 -> [w1679 w1705]
          tunnel: w1676 -> [_ w1701]
          tunnel: w1675 -> [_ w1700]
          tunnel: w1674 -> [_ w1698]
          tunnel: w1673 -> [_ w1697]
          tunnel: w1672 -> [_ w1696]
          tunnel: w1671 -> [_ w1693]
          tunnel: [w1679 w1687] -> w1669
          tunnel: w1668 -> [_ w1685]
          tunnel: w1667 -> [_ w1684]
          tunnel: 2 -> [_ w1680]
          frame False {
          }
          frame True {
            n650 = property class="Ring (严格)"(reference=w1684) -> ("Value"=w1683:u16)  [unwired: 1 in, 2 out]
            n651 = property class="Str"(reference=w1685, "DisabledEnum"=w1680) -> (reference out=w1682:refnum<vi>, "Value"=w1681:string)  [unwired: 1 in, 1 out]
            n652 = property class="Str"(reference=w1696) -> (reference out=w1694:refnum<vi>, "Value"=w1695:string)  [unwired: 1 in, 1 out]
            n653 = property class="Str"(reference=w1693) -> (reference out=w1688:refnum<vi>, "Value"=w1692:string)  [unwired: 1 in, 1 out]
            n654 = Empty String/Path?(string/path=w1695) -> (empty?=w1690:bool)
            n655 = Empty String/Path?(string/path=w1692) -> (empty?=w1691:bool)
            n656 = call "ShipmentClarity.vi"("产品种类"=w1683, "包装箱条码"=w1681, "error in"=w1705, "Debug"=TRUE) -> ("error out"=w1699:errorcluster, "SNStr"=w1702:string, "包装方式"=w1703:u32, "外购？"=w1704:bool)  [unwired: 4 in]
            n657 = Or(x=w1690, y=w1691) -> (x .or. y?=w1689:bool)
            n658 = case shown="假" w1689 {
              tunnel: w1704 -> [w1716 _]
              tunnel: w1703 -> [w1715 _]
              tunnel: w1702 -> [w1714 _]
              tunnel: w1701 -> [w1713 _]
              tunnel: w1700 -> [w1712 _]
              tunnel: w1699 -> [w1711 w1987]
              tunnel: w1698 -> [w1710 _]
              tunnel: w1697 -> [w1709 _]
              tunnel: w1694 -> [_ w1992]
              tunnel: w1688 -> [_ w1991]
              tunnel: [w1708 w1982] -> w1687
              tunnel: w1682 -> [w1706 w1985]
              tunnel: w1681 -> [w1707 _]
              frame False {
                n659 = case shown="真" w1716 {
                  tunnel: w1715 -> [w1731 w1820]
                  tunnel: w1714 -> [w1730 w1819]
                  tunnel: w1713 -> [w1729 w1813]
                  tunnel: w1712 -> [w1722 w1818]
                  tunnel: w1711 -> [w1726 w1817]
                  tunnel: w1710 -> [w1725 w1816]
                  tunnel: w1709 -> [w1720 w1815]
                  tunnel: [w1724 w1811] -> w1708
                  tunnel: w1707 -> [_ w1810]
                  tunnel: w1706 -> [w1718 w1809]
                  frame False {
                    n660 = property class="Str"(reference=w1722) -> ("Value"=w1721:string)  [unwired: 1 in, 2 out]
                    n661 = property class="MCListbox (严格)"(reference=w1729, "ColHdrString"=string[] ["数据ID", "SIM卡号", "SN号", "IMEI", "测试结果", "测试日期", "箱号"]) -> (reference out=w1727:refnum<vi>, "Value"=w1723:i32)  [unwired: 1 in, 1 out]
                    n662 = property class="Str"(reference=w1720) -> (reference out=w1717:refnum<vi>, "Value"=w1719:string)  [unwired: 1 in, 1 out]
                    n663 = case shown="2" w1731 {
                      tunnel: w1730 -> [w1741 _]
                      tunnel: w1727 -> [_ w1760]
                      tunnel: w1722 -> [_ w1759]
                      tunnel: w1726 -> [w1740 w1753]
                      tunnel: w1725 -> [_ w1758]
                      tunnel: [w1733 w1757] -> w1724
                      tunnel: w1723 -> [_ w1756]
                      tunnel: w1721 -> [_ w1755]
                      tunnel: w1719 -> [_ w1754]
                      tunnel: w1718 -> [w1739 w1748]
                      tunnel: w1717 -> [_ w1750]
                      frame 0, Default {
                        n664 = flat-sequence {
                          tunnel: w1741 -> [w1744]
                          tunnel: [w1743] -> _
                          tunnel: w1740 -> [w1742]
                          tunnel: [w1742] -> w1738
                          frame #0 {
                            n665 = Concatenate Strings("箱内有部分产品未走包装程序：", "\n", w1744) -> (w1745:string)
                            n666 = One Button Dialog(message=w1745) -> (true=w1743:bool)  [unwired: 1 in]
                          }
                        }
                        n667 = property class="Str"(reference=w1739, error in=w1738, "Value"="", "DisabledEnum"=0) -> (reference out=w1735:refnum<vi>, error out=w1734:errorcluster)
                        n668 = property class="Str"(reference=w1735, error in=w1734, "Key Focus"=TRUE) -> (error out=w1733:errorcluster)  [unwired: 1 out]
                      }
                      frame 2 {
                        n669 = call "SOutFlagJudge.vi"("error in"=w1753, "包装箱条码"=w1754) -> ("error out"=w1751:errorcluster, "Str"=w1749:string, "OK?"=w1752:bool)  [unwired: 7 in]
                        n670 = case shown="假" w1752 {
                          tunnel: w1760 -> [_ w1786]
                          tunnel: w1759 -> [_ w1785]
                          tunnel: w1758 -> [_ w1784]
                          tunnel: [w1761 w1783] -> w1757
                          tunnel: w1756 -> [_ w1782]
                          tunnel: w1755 -> [_ w1781]
                          tunnel: w1754 -> [_ w1780]
                          tunnel: w1751 -> [w1762 _]
                          tunnel: w1750 -> [w1764 _]
                          tunnel: w1749 -> [w1763 _]
                          tunnel: w1748 -> [_ w1779]
                          frame False {
                            n671 = flat-sequence {
                              tunnel: w1763 -> [w1776]
                              tunnel: w1762 -> [w1774]
                              tunnel: [w1774] -> w1765
                              tunnel: [w1773] -> _
                              tunnel: [w1772] -> w1771
                              tunnel: w1764 -> [w1772]
                              frame #0 {
                                n672 = Concatenate Strings("本箱有部分产品已走出货流程！", "\n", w1776) -> (w1775:string)
                                n673 = One Button Dialog(message=w1775) -> (true=w1773:bool)  [unwired: 1 in]
                              }
                            }
                            n674 = property class="Str"(reference=w1771, error in=w1765, "Value"="", "DisabledEnum"=0) -> (reference out=w1768:refnum<vi>, error out=w1767:errorcluster)
                            n675 = property class="Str"(reference=w1768, error in=w1767, "Key Focus"=TRUE) -> (error out=w1761:errorcluster)  [unwired: 1 out]
                          }
                          frame True {
                            n676 = call "ShipDataJudAndView.vi"("包装箱条码"=w1780, "设定出货数量"=w1781, "箱内产品信息"=w1782, "产品种类"=enum16{"自产", "外购"}."自产", "Debug"=FALSE, "出货数量"=w1785, "箱内产品"=w1786) -> ("error out"=w1788:errorcluster, "AutoShipFlash"=w1789:bool)  [unwired: 3 in]
                            n677 = case shown="假" w1789 {
                              tunnel: w1788 -> [w1792 w1806]
                              tunnel: w1784 -> [_ w1808]
                              tunnel: [w1791 w1805] -> w1783
                              tunnel: w1779 -> [w1793 w1804]
                              frame False {
                                n678 = property class="Str"(reference=w1793, error in=w1792, "Value"="", "DisabledEnum"=0) -> (reference out=w1796:refnum<vi>, error out=w1795:errorcluster)
                                n679 = property class="Str"(reference=w1796, error in=w1795, "Key Focus"=TRUE) -> (error out=w1791:errorcluster)  [unwired: 1 out]
                              }
                              frame True {
                                n680 = property class="Str"(reference=w1804, "Value"="", "DisabledEnum"=0) -> (reference out=w1801:refnum<vi>, error out=w1800:errorcluster)  [unwired: 1 in]
                                n681 = property class="Str"(reference=w1801, error in=w1800, "Key Focus"=FALSE) -> ()  [unwired: 2 out]
                                n682 = Generate User Event(user event=w1808, event data cluster="ShipOut" ("事件数据"), error in=w1806) -> (error out=w1805:errorcluster)  [unwired: 1 in, 1 out]
                              }
                            }
                          }
                        }
                      }
                    }
                  }
                  frame True {
                    n683 = property class="MCListbox (严格)"(reference=w1813, "ColHdrString"=string[] ["数据ID", "型号", "SIM卡号", "ICCID号", "SN号", "导入日期", "箱号"]) -> (reference out=w1814:refnum<vi>)  [unwired: 1 in, 1 out]
                    n684 = case shown="2" w1820 {
                      tunnel: w1819 -> [w1826 _ _]
                      tunnel: w1814 -> [_ w1853 w1922]
                      tunnel: w1818 -> [_ w1852 w1921]
                      tunnel: w1817 -> [w1822 w1847 w1915]
                      tunnel: w1816 -> [_ w1851 w1920]
                      tunnel: w1815 -> [_ w1848 w1919]
                      tunnel: [w1821 w1850 w1918] -> w1811
                      tunnel: w1810 -> [_ w1849 w1917]
                      tunnel: w1809 -> [w1825 _ w1916]
                      frame 0, Default {
                        n685 = flat-sequence {
                          tunnel: w1826 -> [w1830]
                          tunnel: w1825 -> [w1828]
                          tunnel: [w1828] -> w1824
                          tunnel: [w1827] -> w1823
                          tunnel: w1822 -> [w1827]
                          tunnel: w1824 -> [w1840]
                          tunnel: [w1834] -> w1821
                          tunnel: w1823 -> [w1833]
                          frame #0 {
                            n686 = Concatenate Strings("箱内有部分产品未走包装程序：", "\n", w1830) -> (w1829:string)
                            n687 = One Button Dialog(message=w1829) -> ()  [unwired: 1 in, 1 out]
                          }
                          frame #1 {
                            n688 = property class="Str"(reference=w1840, error in=w1833, "Value"="", "DisabledEnum"=0) -> (reference out=w1836:refnum<vi>, error out=w1837:errorcluster)
                            n689 = property class="Str"(reference=w1836, error in=w1837, "Key Focus"=TRUE) -> (error out=w1834:errorcluster)  [unwired: 1 out]
                          }
                        }
                      }
                      frame 2 {
                        n690 = property class="Str"(reference=w1848, error in=w1847) -> (reference out=w1844:refnum<vi>, error out=w1846:errorcluster, "Value"=w1841:string)
                        n691 = call "OutFlagJudge.vi"("error in"=w1846, "包装箱条码"=w1841) -> ("error out"=w1842:errorcluster, "Str"=w1843:string, "OK?"=w1845:bool)  [unwired: 7 in]
                        n692 = case shown="真" w1845 {
                          tunnel: w1853 -> [_ w1875]
                          tunnel: w1852 -> [_ w1874]
                          tunnel: w1851 -> [_ w1873]
                          tunnel: [w1854 w1880] -> w1850
                          tunnel: w1849 -> [_ w1872]
                          tunnel: w1844 -> [w1857 w1876]
                          tunnel: w1843 -> [w1856 _]
                          tunnel: w1842 -> [w1855 w1878]
                          tunnel: w1841 -> [_ w1881]
                          frame False {
                            n693 = flat-sequence {
                              tunnel: w1856 -> [w1869]
                              tunnel: w1855 -> [w1867]
                              tunnel: [w1867] -> w1858
                              tunnel: [w1866] -> _
                              tunnel: [w1865] -> w1864
                              tunnel: w1857 -> [w1865]
                              frame #0 {
                                n694 = Concatenate Strings("本箱有部分产品已走出货流程！", "\n", w1869) -> (w1868:string)
                                n695 = One Button Dialog(message=w1868) -> (true=w1866:bool)  [unwired: 1 in]
                              }
                            }
                            n696 = property class="Str"(reference=w1864, error in=w1858, "Value"="", "DisabledEnum"=0) -> (reference out=w1861:refnum<vi>, error out=w1860:errorcluster)
                            n697 = property class="Str"(reference=w1861, error in=w1860, "Key Focus"=TRUE) -> (error out=w1854:errorcluster)  [unwired: 1 out]
                          }
                          frame True {
                            n698 = call "BSJShipPackage.vi"("error in"=w1878, "包装箱条码"=w1881) -> ("error out"=w1877:errorcluster, "OK？"=w1879:bool)  [unwired: 8 in]
                            n699 = case shown="真" w1879 {
                              tunnel: [w1882 w1890] -> w1880
                              tunnel: w1877 -> [w1882 w1888]
                              tunnel: w1876 -> [_ w1887]
                              tunnel: w1875 -> [_ w1886]
                              tunnel: w1874 -> [_ w1885]
                              tunnel: w1873 -> [_ w1884]
                              tunnel: w1872 -> [_ w1883]
                              frame False {
                              }
                              frame True {
                                n700 = call "ShipDataJudAndView.vi"("包装箱条码"=w1883, "产品种类"=enum16{"自产", "外购"}."外购", "error in"=w1888, "Debug"=FALSE, "出货数量"=w1885, "箱内产品"=w1886) -> ("error out"=w1891:errorcluster, "AutoShipFlash"=w1892:bool)  [unwired: 4 in]
                                n701 = case shown="假" w1892 {
                                tunnel: w1891 -> [w1899 w1908]
                                tunnel: [w1899 w1907] -> w1890
                                tunnel: w1887 -> [w1894 w1901]
                                tunnel: w1884 -> [_ w1900]
                                frame False {
                                n702 = property class="Str"(reference=w1894, "Value"="", "DisabledEnum"=0) -> (reference out=w1896:refnum<vi>)  [unwired: 1 in, 1 out]
                                n703 = property class="Str"(reference=w1896, "Key Focus"=TRUE) -> ()  [unwired: 1 in, 2 out]
                                }
                                frame True {
                                n704 = property class="Str"(reference=w1901, "Value"="", "DisabledEnum"=0) -> (reference out=w1904:refnum<vi>, error out=w1903:errorcluster)  [unwired: 1 in]
                                n705 = Generate User Event(user event=w1900, event data cluster="ShipOut" ("事件数据"), error in=w1908) -> (error out=w1907:errorcluster)  [unwired: 1 in, 1 out]
                                n706 = property class="Str"(reference=w1904, error in=w1903, "Key Focus"=FALSE) -> ()  [unwired: 2 out]
                                }
                                }
                              }
                            }
                          }
                        }
                      }
                      frame 1 {
                        n707 = property class="Str"(reference=w1919) -> (reference out=w1911:refnum<vi>, "Value"=w1910:string)  [unwired: 1 in, 1 out]
                        n708 = call "OutFlagJudge.vi"("error in"=w1915, "包装箱条码"=w1910) -> ("error out"=w1914:errorcluster, "Str"=w1912:string, "OK?"=w1913:bool)  [unwired: 7 in]
                        n709 = case shown="真" w1913 {
                          tunnel: w1922 -> [_ w1950]
                          tunnel: w1921 -> [_ w1949]
                          tunnel: w1914 -> [w1932 w1943]
                          tunnel: w1920 -> [_ w1948]
                          tunnel: [w1925 w1947] -> w1918
                          tunnel: w1917 -> [_ w1946]
                          tunnel: w1916 -> [_ w1945]
                          tunnel: w1912 -> [w1933 _]
                          tunnel: w1911 -> [w1931 _]
                          tunnel: w1910 -> [_ w1944]
                          frame False {
                            n710 = flat-sequence {
                              tunnel: w1933 -> [w1938]
                              tunnel: w1932 -> [w1936]
                              tunnel: [w1936] -> w1923
                              tunnel: [w1935] -> _
                              tunnel: [w1934] -> w1930
                              tunnel: w1931 -> [w1934]
                              frame #0 {
                                n711 = Concatenate Strings("本箱有部分产品已走出货流程！", "\n", w1938) -> (w1937:string)
                                n712 = One Button Dialog(message=w1937) -> (true=w1935:bool)  [unwired: 1 in]
                              }
                            }
                            n713 = property class="Str"(reference=w1930, error in=w1923, "Value"="", "DisabledEnum"=0) -> (reference out=w1927:refnum<vi>, error out=w1926:errorcluster)
                            n714 = property class="Str"(reference=w1927, error in=w1926, "Key Focus"=TRUE) -> (error out=w1925:errorcluster)  [unwired: 1 out]
                          }
                          frame True {
                            n715 = call "BSJShipPackage.vi"("error in"=w1943, "包装箱条码"=w1944) -> ("error out"=w1941:errorcluster, "OK？"=w1942:bool)  [unwired: 8 in]
                            n716 = case shown="真" w1942 {
                              tunnel: w1950 -> [_ w1962]
                              tunnel: w1949 -> [_ w1961]
                              tunnel: w1948 -> [_ w1957]
                              tunnel: [w1951 w1956] -> w1947
                              tunnel: w1946 -> [_ w1955]
                              tunnel: w1945 -> [_ w1953]
                              tunnel: w1941 -> [w1951 w1952]
                              frame False {
                              }
                              frame True {
                                n717 = call "ShipDataJudAndView.vi"("包装箱条码"=w1955, "产品种类"=enum16{"自产", "外购"}."外购", "error in"=w1952, "Debug"=FALSE, "出货数量"=w1961, "箱内产品"=w1962) -> ("error out"=w1958:errorcluster, "AutoShipFlash"=w1959:bool)  [unwired: 4 in]
                                n718 = case shown="假" w1959 {
                                tunnel: w1958 -> [w1965 w1972]
                                tunnel: w1957 -> [_ w1981]
                                tunnel: [w1964 w1979] -> w1956
                                tunnel: w1953 -> [w1970 w1978]
                                frame False {
                                n719 = property class="Str"(reference=w1970, error in=w1965, "Value"="", "DisabledEnum"=0) -> (reference out=w1967:refnum<vi>, error out=w1963:errorcluster)
                                n720 = property class="Str"(reference=w1967, error in=w1963, "Key Focus"=TRUE) -> (error out=w1964:errorcluster)  [unwired: 1 out]
                                }
                                frame True {
                                n721 = property class="Str"(reference=w1978, error in=w1972, "Value"="", "DisabledEnum"=0) -> (reference out=w1975:refnum<vi>, error out=w1974:errorcluster)
                                n722 = property class="Str"(reference=w1975, error in=w1974, "Key Focus"=FALSE) -> (error out=w1971:errorcluster)  [unwired: 1 out]
                                n723 = Generate User Event(user event=w1981, event data cluster="ShipOut" ("事件数据"), error in=w1971) -> (error out=w1979:errorcluster)  [unwired: 1 in, 1 out]
                                }
                                }
                              }
                            }
                          }
                        }
                      }
                    }
                  }
                }
              }
              frame True {
                n724 = flat-sequence {
                  tunnel: w1992 -> [w1999]
                  tunnel: [w1999] -> w1990
                  tunnel: w1991 -> [w1998]
                  tunnel: [w1998] -> w1989
                  tunnel: [w1997] -> _
                  frame #0 {
                    n725 = One Button Dialog(message="出货地址或出货数量为空！\n请先输入正确的出货地址和数量！" ("消息")) -> (true=w1997:bool)  [unwired: 1 in]
                  }
                }
                n726 = Build Array(w1990, w1989) -> (w1988:refnum<vi>[])
                n727 = for {
                  tunnel: w1988 -> [w1996] mode=indexing
                  tunnel: w1987 -> [w1994]
                  tunnel: [w1993] -> w1986
                  n728 = property class="Str"(reference=w1996, error in=w1994, "DisabledEnum"=0) -> (error out=w1993:errorcluster)  [unwired: 1 out]
                }
                n729 = property class="Str"(reference=w1985, error in=w1986, "Value"="" ("值"), "DisabledEnum"=0) -> (error out=w1982:errorcluster)  [unwired: 1 out]
              }
            }
          }
        }
      }
      event User Event {
        n730 = event-data() -> ("ExportEve"=w2008:string)  [unwired: 1 in]
        n731 = case shown="\"假\", 默认" w2008 {
          tunnel: w2007 -> [_ w2036]
          tunnel: w2006 -> [_ w2032]
          tunnel: w2005 -> [_ w2021]
          tunnel: w2003 -> [w2009 w2012]
          tunnel: [w2009 w2011] -> w2002
          tunnel: w2001 -> [_ w2010]
          frame "假", Default {
          }
          frame "ShipOut" {
            n732 = property class="MCListbox (严格)"(reference=w2036, error in=w2012) -> (reference out=w2023:refnum<vi>, error out=w2028:errorcluster, "ItemNames"=w2035:string[][])
            n733 = Unbundle By Name(w2021) -> ("产品种类"=w2020:refnum<vi>)
            n734 = property class="Str"(reference=w2032) -> ("Value"=w2030:string)  [unwired: 1 in, 2 out]
            n735 = property class="Ring (严格)"(reference=w2020) -> ("RingText.Text"=w2019:string)  [unwired: 1 in, 2 out]
            n736 = Index Array(array=w2035, index (col)=6) -> (element=w2033:string[])  [unwired: 1 in]
            n737 = Match Pattern(string=w2019, regular expression="外购" ("正则表达式")) -> (offset past match=w2017:i32)  [unwired: 1 in, 3 out]
            n738 = call "ArrayFilter.vi"("error in"=w2028, "ArrayIn"=w2033) -> ("error out"=w2029:errorcluster, "ArrayOut"=w2031:string[])  [unwired: 8 in]
            n739 = Greater Or Equal To 0?(x=w2017) -> (x >= 0?=w2016:bool)
            n740 = case shown="真" w2016 {
              tunnel: ["prc_MFlashAdress" ("SQL query") "prc_BSJFlashAdress" ("SQL query")] -> w2015
              frame False {
              }
              frame True {
              }
            }
            n741 = for {
              tunnel: w2031 -> [w2079] mode=indexing
              tunnel: w2030 -> [w2078]
              tunnel: w2029 -> [w2073]
              tunnel: [w2072] -> w2022
              tunnel: [w2067] -> w2026 mode=indexing
              tunnel: w2015 -> [w2069]
              tunnel: [w2067] -> w2014 mode=indexing if=w2066
              w2076 = ","
              w2077 = "'"
              n742 = Concatenate Strings(w2077, w2079, w2077, w2076, w2077, w2078, w2077, w2076, "@A" ("字符串")) -> (w2074:string)
              n743 = call "prc_SetPackaged.vi"("error in"=w2073, "string"=w2074, "SQL query"=w2069) -> ("error out"=w2072:errorcluster, "Array"=w2071:string[][])  [unwired: 7 in]
              n744 = Index Array(array=w2071) -> (element=w2070:string[])  [unwired: 2 in]
              n745 = Index Array(array=w2070) -> (element=w2067:string)  [unwired: 1 in]
              n746 = Not Equal?(x="OK" ("字符串"), y=w2067) -> (x != y?=w2066:bool)
            }
            n747 = Index Array(array=w2014) -> (element=w2013:string)  [unwired: 1 in]
            n748 = Equal?(x=w2026, y="OK" ("字符串")) -> (x = y?=w2025:bool[])
            n749 = And Array Elements(Boolean array=w2025) -> (logical AND=w2024:bool)
            n750 = case shown="假" w2024 {
              tunnel: w2023 -> [_ w2062]
              tunnel: w2022 -> [w2045 w2056]
              tunnel: w2021 -> [_ w2055]
              tunnel: w2013 -> [w2048 _]
              tunnel: [w2040 w2051] -> w2011
              tunnel: w2010 -> [w2047 _]
              frame False {
                n751 = flat-sequence {
                  tunnel: w2048 -> [w2050]
                  tunnel: [w2049] -> w2046
                  tunnel: w2045 -> [w2049]
                  frame #0 {
                    n752 = One Button Dialog(message=w2050) -> ()  [unwired: 1 in, 1 out]
                  }
                }
                n753 = property class="Str"(reference=w2047, error in=w2046, "Value"="", "DisabledEnum"=0) -> (reference out=w2042:refnum<vi>, error out=w2041:errorcluster)
                n754 = property class="Str"(reference=w2042, error in=w2041, "Key Focus"=TRUE) -> (error out=w2040:errorcluster)  [unwired: 1 out]
              }
              frame True {
                n755 = Unbundle By Name(w2055) -> ("设定出货数量"=w2053:refnum<vi>, "出货地址"=w2052:refnum<vi>)
                n756 = invoke class="MCListbox (严格)" method="Reinit To Default"(reference=w2062, error in=w2056) -> (reference out=w2061:refnum<vi>, error out=w2060:errorcluster)  [unwired: 1 in, 1 out]
                n757 = Build Array(w2053, w2052) -> (w2054:refnum<vi>[])
                n758 = for {
                  tunnel: w2054 -> [w2065] mode=indexing
                  n759 = property class="Str"(reference=w2065, "Value"="", "DisabledEnum"=0) -> ()  [unwired: 1 in, 2 out]
                }
                n760 = property class="MCListbox (严格)"(reference=w2061, error in=w2060, "SelColor"=u32 16775631, "RowHdrs[]"=string[] [] ("行首字符串[]"), "ItemNames"=string[][] [] ("项名")) -> (error out=w2051:errorcluster)  [unwired: 1 out]
              }
            }
          }
        }
      }
      event "手动出货": Value Change {
        n761 = event-data() -> ("CtlRef"=w2085:refnum<vi>, "NewVal"=w2088:bool)  [unwired: 1 in]
        n762 = property class="MCListbox (严格)"(reference=w2090, error in=w2081) -> (error out=w2083:errorcluster, "ItemNames"=w2089:string[][])  [unwired: 1 out]
        n763 = case shown="真" w2088 {
          tunnel: [w2092 w2100] -> w2091
          tunnel: w2089 -> [_ w2099]
          tunnel: w2087 -> [_ w2096]
          tunnel: [w2093 w2095] -> w2086
          tunnel: w2085 -> [w2093 w2095]
          tunnel: w2083 -> [w2092 w2094]
          frame False {
          }
          frame True {
            n764 = Array Size(array=w2099) -> (size(s)=w2098:i32[])
            n765 = Index Array(array=w2098) -> (element=w2097:i32)  [unwired: 1 in]
            n766 = Greater Or Equal?(x=w2097, y=1) -> (x >= y?=w2101:bool)
            n767 = case shown="真" w2101 {
              tunnel: [w2103 w2107] -> w2100
              tunnel: w2096 -> [_ w2106]
              tunnel: w2094 -> [w2103 w2105]
              frame False {
                n768 = One Button Dialog(message="包装箱为空！" ("消息")) -> ()  [unwired: 1 in, 1 out]
              }
              frame True {
                n769 = Generate User Event(user event=w2106, event data cluster="ShipOut" ("事件数据"), error in=w2105) -> (error out=w2107:errorcluster)  [unwired: 1 in, 1 out]
              }
            }
          }
        }
        n770 = property class="Bool (严格)"(reference=w2086, error in=w2091, "Value"=FALSE ("值")) -> (error out=w2080:errorcluster)  [unwired: 1 out]
      }
      event "开始时间", "结束时间", "导出方式", "型号": Value Change {
        n771 = event-data() -> ()  [unwired: 1 in, 2 out]
        n772 = property class="Ring (严格)"(reference=w2112, error in=w2111) -> (error out=w2110:errorcluster, "Value"=w2109:u16)  [unwired: 1 out]
        n773 = case shown="0, 2" w2109 {
          frame 1, Default {
          }
          frame 0, 2 {
          }
        }
      }
      event "导出": Value Change {
        n774 = event-data() -> ("CtlRef"=w2115:refnum<vi>)  [unwired: 1 in]
        n775 = property class="Ring (严格)"(reference=w2126) -> ("RingText.Text"=w2124:string)  [unwired: 1 in, 2 out]
        n776 = Unbundle By Name(w2120) -> ("导出方式"=w2116:refnum<vi>, "开始时间"=w2119:refnum<vi>, "结束时间"=w2118:refnum<vi>, "地址"=w2117:refnum<vi>)
        n777 = Match Pattern(string=w2124, regular expression="外购" ("正则表达式")) -> (offset past match=w2122:i32)  [unwired: 1 in, 3 out]
        n778 = Greater Or Equal To 0?(x=w2122) -> (x >= 0?=w2121:bool)
        n779 = case shown="假" w2121 {
          tunnel: w2125 -> [w2144 w2206]
          tunnel: w2119 -> [w2142 w2204]
          tunnel: w2118 -> [w2140 w2202]
          tunnel: w2117 -> [w2137 w2199]
          tunnel: w2116 -> [w2135 w2197]
          tunnel: w2115 -> [w2133 w2195]
          tunnel: w2114 -> [w2130 w2193]
          tunnel: [w2131 w2191] -> w2113
          frame True {
            w2138 = "%Y-%m-%d %H:%M:%S"
            n780 = property class="AbsTime (严格)"(reference=w2142) -> ("Value"=w2141:timestamp)  [unwired: 1 in, 2 out]
            n781 = property class="AbsTime (严格)"(reference=w2140) -> ("Value"=w2139:timestamp)  [unwired: 1 in, 2 out]
            n782 = property class="Ring (严格)"(reference=w2135, error in=w2130) -> (error out=w2129:errorcluster, "RingText.Text"=w2134:string)  [unwired: 1 out]
            n783 = property class="Ring (严格)"(reference=w2144) -> ("RingText.Text"=w2143:string)  [unwired: 1 in, 2 out]
            n784 = property class="Str"(reference=w2137) -> ("Value"=w2136:string)  [unwired: 1 in, 2 out]
            n785 = Format Date/Time String(time format string (%c)=w2138, seconds (now)=w2141) -> (date/time string=w2162:string)  [unwired: 1 in]
            n786 = Format Date/Time String(time format string (%c)=w2138, seconds (now)=w2139) -> (date/time string=w2161:string)  [unwired: 1 in]
            n787 = call <vilib>:"Application Directory.vi"() -> ("Application Directory"=w2157:path)
            n788 = Build Array(w2143, w2162, w2161, w2134, w2136) -> (w2163:string[])
            n789 = Build Path(base path=w2157, name or relative path="Result" ("数据 2")) -> (appended path=w2155:path)
            n790 = for {
              tunnel: w2163 -> [w2188] mode=indexing
              shift-right: [w2189] -> w2159
              shift-left: "" -> [w2190]
              w2187 = "'" ("字符串")
              n791 = Concatenate Strings(w2190, w2187, w2188, w2187, "," ("字符串")) -> (w2189:string)
            }
            n792 = call <vilib>:"Check if File or Folder Exists.vi"("path"=w2155) -> ("file or folder exists?"=w2154:bool, "dup path"=w2153:path)  [unwired: 8 in, 1 out]
            n793 = case shown="假" w2154 {
              tunnel: w2153 -> [w2166 w2167]
              tunnel: [w2165 w2167] -> w2152
              frame False {
                n794 = Create Folder(path (use dialog)=w2166) -> (created path=w2165:path)  [unwired: 2 in, 2 out]
              }
              frame True {
              }
            }
            n795 = Format Date/Time String(time format string (%c)="BSJ%Y-%m-%d %H%M%S" ("时间格式字符串(%c)")) -> (date/time string=w2150:string)  [unwired: 2 in]
            n796 = Concatenate Strings(w2150, ".xls" ("字符串")) -> (w2148:string)
            n797 = Concatenate Strings(w2159, "@A" ("字符串")) -> (w2158:string)
            n798 = Build Path(base path=w2152, name or relative path=w2148) -> (appended path=w2147:path)
            n799 = call "Get Need data.vi"("error in"=w2129, "string"=w2158, "Procedure"="prc_BSJExportData") -> ("error out"=w2128:errorcluster, "Array"=w2146:string[][])  [unwired: 7 in]
            n800 = flat-sequence {
              tunnel: w2147 -> [w2173]
              tunnel: w2146 -> [w2174]
              tunnel: w2133 -> [w2171]
              tunnel: string[] ["产品型号", "SIM码", "ICCID号", "SN号", "发货地址", "包装时间"] -> [w2170]
              tunnel: [w2169] -> w2131
              tunnel: w2128 -> [w2168]
              frame #0 {
                n801 = case shown="假" TRUE {
                  tunnel: w2174 -> [_ w2185]
                  tunnel: w2173 -> [_ w2180]
                  tunnel: [w2176 w2179] -> w2169
                  tunnel: w2170 -> [_ w2178]
                  tunnel: w2168 -> [w2176 w2177]
                  frame False {
                  }
                  frame True {
                    n802 = Insert Into Array(array=w2185, index (row)=0 ("索引 (行)"), new element=w2178) -> (w2183:string[][])  [unwired: 1 in]
                    n803 = call "TableStrAdd.vi"("error in"=w2177, "Array"=w2183) -> ("error out"=w2181:errorcluster, "数组"=w2182:string[][])
                    n804 = call "ReportProcess.vi"("error in"=w2181, "text data"=w2182, "Path"=w2180) -> ("error out"=w2179:errorcluster)  [unwired: 8 in]
                  }
                }
                n805 = property class="Bool (严格)"(reference=w2171, "Value"=FALSE) -> ()  [unwired: 1 in, 2 out]
              }
            }
          }
          frame False {
            w2200 = "%Y-%m-%d %H:%M:%S"
            n806 = property class="AbsTime (严格)"(reference=w2204) -> ("Value"=w2203:timestamp)  [unwired: 1 in, 2 out]
            n807 = property class="AbsTime (严格)"(reference=w2202) -> ("Value"=w2201:timestamp)  [unwired: 1 in, 2 out]
            n808 = property class="Ring (严格)"(reference=w2197) -> ("RingText.Text"=w2196:string)  [unwired: 1 in, 2 out]
            n809 = property class="Ring (严格)"(reference=w2206) -> ("RingText.Text"=w2205:string)  [unwired: 1 in, 2 out]
            n810 = property class="Str"(reference=w2199) -> ("Value"=w2198:string)  [unwired: 1 in, 2 out]
            n811 = Format Date/Time String(time format string (%c)=w2200, seconds (now)=w2203) -> (date/time string=w2224:string)  [unwired: 1 in]
            n812 = Format Date/Time String(time format string (%c)=w2200, seconds (now)=w2201) -> (date/time string=w2223:string)  [unwired: 1 in]
            n813 = call <vilib>:"Application Directory.vi"() -> ("Application Directory"=w2219:path)
            n814 = Build Array(w2205, w2224, w2223, w2196, w2198) -> (w2225:string[])
            n815 = Build Path(base path=w2219, name or relative path="Result" ("数据 2")) -> (appended path=w2217:path)
            n816 = for {
              tunnel: w2225 -> [w2250] mode=indexing
              shift-right: [w2251] -> w2221
              shift-left: "" -> [w2252]
              w2249 = "'" ("字符串")
              n817 = Concatenate Strings(w2252, w2249, w2250, w2249, "," ("字符串")) -> (w2251:string)
            }
            n818 = call <vilib>:"Check if File or Folder Exists.vi"("path"=w2217) -> ("file or folder exists?"=w2216:bool, "dup path"=w2215:path)  [unwired: 8 in, 1 out]
            n819 = case shown="假" w2216 {
              tunnel: w2215 -> [w2228 w2229]
              tunnel: [w2227 w2229] -> w2214
              frame False {
                n820 = Create Folder(path (use dialog)=w2228) -> (created path=w2227:path)  [unwired: 2 in, 2 out]
              }
              frame True {
              }
            }
            n821 = Format Date/Time String(time format string (%c)="ZC%Y-%m-%d %H%M%S" ("时间格式字符串(%c)")) -> (date/time string=w2212:string)  [unwired: 2 in]
            n822 = Concatenate Strings(w2212, ".xls" ("字符串")) -> (w2210:string)
            n823 = Concatenate Strings(w2221, "@A" ("字符串")) -> (w2220:string)
            n824 = Build Path(base path=w2214, name or relative path=w2210) -> (appended path=w2209:path)
            n825 = call "Get Need data.vi"("error in"=w2193, "string"=w2220, "Procedure"="prc_MExportData") -> ("error out"=w2192:errorcluster, "Array"=w2208:string[][])  [unwired: 7 in]
            n826 = flat-sequence {
              tunnel: w2209 -> [w2235]
              tunnel: w2208 -> [w2236]
              tunnel: [w2234] -> w2191
              tunnel: w2195 -> [w2232]
              tunnel: string[] ["终端ID", "SN码", "发货地址", "CCID号", "软件版本", "测试日期"] -> [w2231]
              tunnel: w2192 -> [w2230]
              frame #0 {
                n827 = case shown="真" TRUE {
                  tunnel: w2236 -> [_ w2247]
                  tunnel: w2235 -> [_ w2242]
                  tunnel: [w2238 w2241] -> w2234
                  tunnel: w2231 -> [_ w2240]
                  tunnel: w2230 -> [w2238 w2239]
                  frame False {
                  }
                  frame True {
                    n828 = Insert Into Array(array=w2247, index (row)=0 ("索引 (行)"), new element=w2240) -> (w2245:string[][])  [unwired: 1 in]
                    n829 = call "TableStrAdd.vi"("error in"=w2239, "Array"=w2245) -> ("error out"=w2243:errorcluster, "数组"=w2244:string[][])
                    n830 = call "ReportProcess.vi"("error in"=w2243, "text data"=w2244, "Path"=w2242) -> ("error out"=w2241:errorcluster)  [unwired: 8 in]
                  }
                }
                n831 = property class="Bool (严格)"(reference=w2232, "Value"=FALSE) -> ()  [unwired: 1 in, 2 out]
              }
            }
          }
        }
      }
    }
  }
  n832 = Unregister For Events(event registration refnum=w23, error in=w19) -> (error out=w14:errorcluster)
  n833 = Unregister For Events(event registration refnum=w24, error in=w20) -> (error out=w16:errorcluster)
  n834 = Unregister For Events(event registration refnum=w25, error in=w21) -> (error out=w18:errorcluster)
  n835 = Destroy User Event(user event=w15, error in=w16) -> (error out=w11:errorcluster)
  n836 = Destroy User Event(user event=w13, error in=w14) -> (error out=w10:errorcluster)
  n837 = Destroy User Event(user event=w17, error in=w18) -> (error out=w12:errorcluster)
  n838 = Merge Errors(w12, w11, w10) -> (w9:errorcluster)
  n839 = flat-sequence {
    tunnel: w9 -> [w2254]
    tunnel: [w2257] -> _
    tunnel: w3 -> [w2256]
    frame #0 {
      n840 = property class="App"(error in=w2254) -> (error out=w2258:errorcluster, "App.Kind"=w2259:T5)  [unwired: 1 in, 1 out]
      n841 = flat-sequence {
        tunnel: w2256 -> [w2262]
        tunnel: [w2262] -> w2255
        tunnel: w2254 -> [w2261]
        tunnel: [w2260] -> w2253
        tunnel: w2255 -> [w2272]
        tunnel: w2253 -> [_]
        frame #0 {
          n842 = call <vilib>:"Clear Errors.vi"("error in (no error)"=w2261) -> ("error out"=w2260:errorcluster)  [unwired: 6 in]
        }
        frame #1 {
          n843 = Unbundle By Name(w2272) -> ("设定大箱总数"=w2271:refnum<vi>, "条码"=w2270:refnum<vi>, "出货地址"=w2268:refnum<vi>, "设定出货数量"=w2267:refnum<vi>, "包装箱条码"=w2266:refnum<vi>, "产品条码"=w2265:refnum<vi>, "SN码"=w2264:refnum<vi>)
          n844 = Build Array(w2270, w2268, w2267, w2266, w2265, w2264) -> (w2269:refnum<vi>[])
          n845 = property class="DigNum (严格)"(reference=w2271, "DisabledEnum"=0) -> ()  [unwired: 1 in, 2 out]
          n846 = for {
            tunnel: w2269 -> [w2274] mode=indexing
            n847 = property class="Str"(reference=w2274, "DisabledEnum"=0) -> ()  [unwired: 1 in, 2 out]
          }
        }
      }
      n848 = case shown="\"Run Time System\"" w2259 {
        tunnel: w2258 -> [w2275 w2276 w2278]
        tunnel: [w2275 w2276 w2277] -> w2257
        frame "invalid app kind", Default {
        }
        frame "Development System" {
        }
        frame "Run Time System" {
          n849 = invoke class="VI" method="FP.Close"(error in=w2278) -> (error out=w2277:errorcluster)  [unwired: 2 in, 2 out]
        }
      }
    }
  }
